vi "总磷总氮通讯.vi"() -> ()   [LabVIEW 2022 SP3, in "斯坦道氨氮.lvlib"]
uses:
  <vilib>/Plasmionique/MB Master/MB_Master_Serial/MB_Master_Serial.lvclass
  C:/Program Files (x86)/National Instruments/LabVIEW 2022/vi.lib/Plasmionique/MB Master/MB_Master/MB_Master.lvclass
  <vilib>/Plasmionique/MB Master/MB_Master_TCP/MB_Master_TCP.lvclass
  <vilib>/Utility/config.llb/Write Key (Boolean).vi
  <vilib>/Utility/config.llb/Write Key (String).vi
  <vilib>/Plasmionique/MB Master/MB_Master/MB_Master.lvclass
  <vilib>/Utility/config.llb/NI_LVConfig.lvlib
  <vilib>/Plasmionique/MB Master/MB Master.lvlib
  <vilib>/ptbypt/NI_PtbyPt.lvlib
panel:
  out "启用":bool=TRUE
  out "氨氮状态告警区":u16[](array[numeric])
  out "氨氮测量数据区":u16[](array[numeric])
  out "COD测量数据区":u16[](array[numeric])
  out "COD状态告警区":u16[](array[numeric])
  out "总氮测量数据区":u16[](array[numeric])
  out "总氮状态告警区":u16[](array[numeric])
  out "总磷状态告警区":u16[](array[numeric])
  out "总磷测量数据区":u16[](array[numeric])
  out "状态告警区":T1 {"告警代码" items=["无告警", "缺试剂告警", "缺水样告警", "缺蒸馏水告警", "缺标液告警", "仪表漏液告警", "标定异常告警", "超量程告警", "加热异常", "低试剂预警", "超上限告警", "超下限告警", "仪表内部其他异常", "滴定异常告警", "电极异常告警", "量程切换告警", "参数设置告警", "PH电极电位异常", "电导率电极异常", "浊度光度异常", "溶解氧电极异常", "溶解氧光强异常", "温度异常告警", "PH异常告警", "溶解氧异常告警", "电导率异常告警", "浊度异常告警", "叶绿素异常告警", "藻密度异常告警", "蓝绿藻异常告警", "ORP异常告警", "氨氮异常告警", "清洁刷异常告警", "SD卡异常告警", "蓝牙异常告警", "Wifi异常告警", "流程异常告警"]; "故障代码" items=["无故障", "电机故障", "温度故障", "通讯故障", "滴定故障"]}
  out "测量数据区":T2 {"单位" items=["ug/L", "mg/L", "ppm", "mg/m3", "cm", "ppb", "ug/m3", "%", "nmol/mol", "umol/mol", "MPN/L", "MPN/100ml", "ng/m3", "NTU", "无量纲", "ms/cm", "us/cm", "℃", "mV", "万个/L"]}
  out "status":bool
  out "关键参数区":T3
  in  "读关键参数区":bool
  in  "读状态告警区":bool
  in  "读测量数据区":bool
  in  "站号":u16(ring) items=["总磷"=1, "氨氮"=3]
  in  "停止":bool
  in  "启动":bool
  in  "控制命令":u16(ring) items=["启动测量"=1, "标样核查"=2, "零点核查"=3, "跨度核查"=4, "空白测试"=5, "平行样测试"=6, "加标回收"=7, "空白校准"=8, "标样校准"=9, "初始化（清洗）"=10, "停止测试"=11, "仪器重启"=12, "校时"=13, "模式设置"=14, "测量间隔设置"=15]
  in  "控制命令参数":u16[](array[numeric]) format="%04xH"
  in  "VISA Resource":refnum<visa-resource-name>
  in  "启用模块":bool
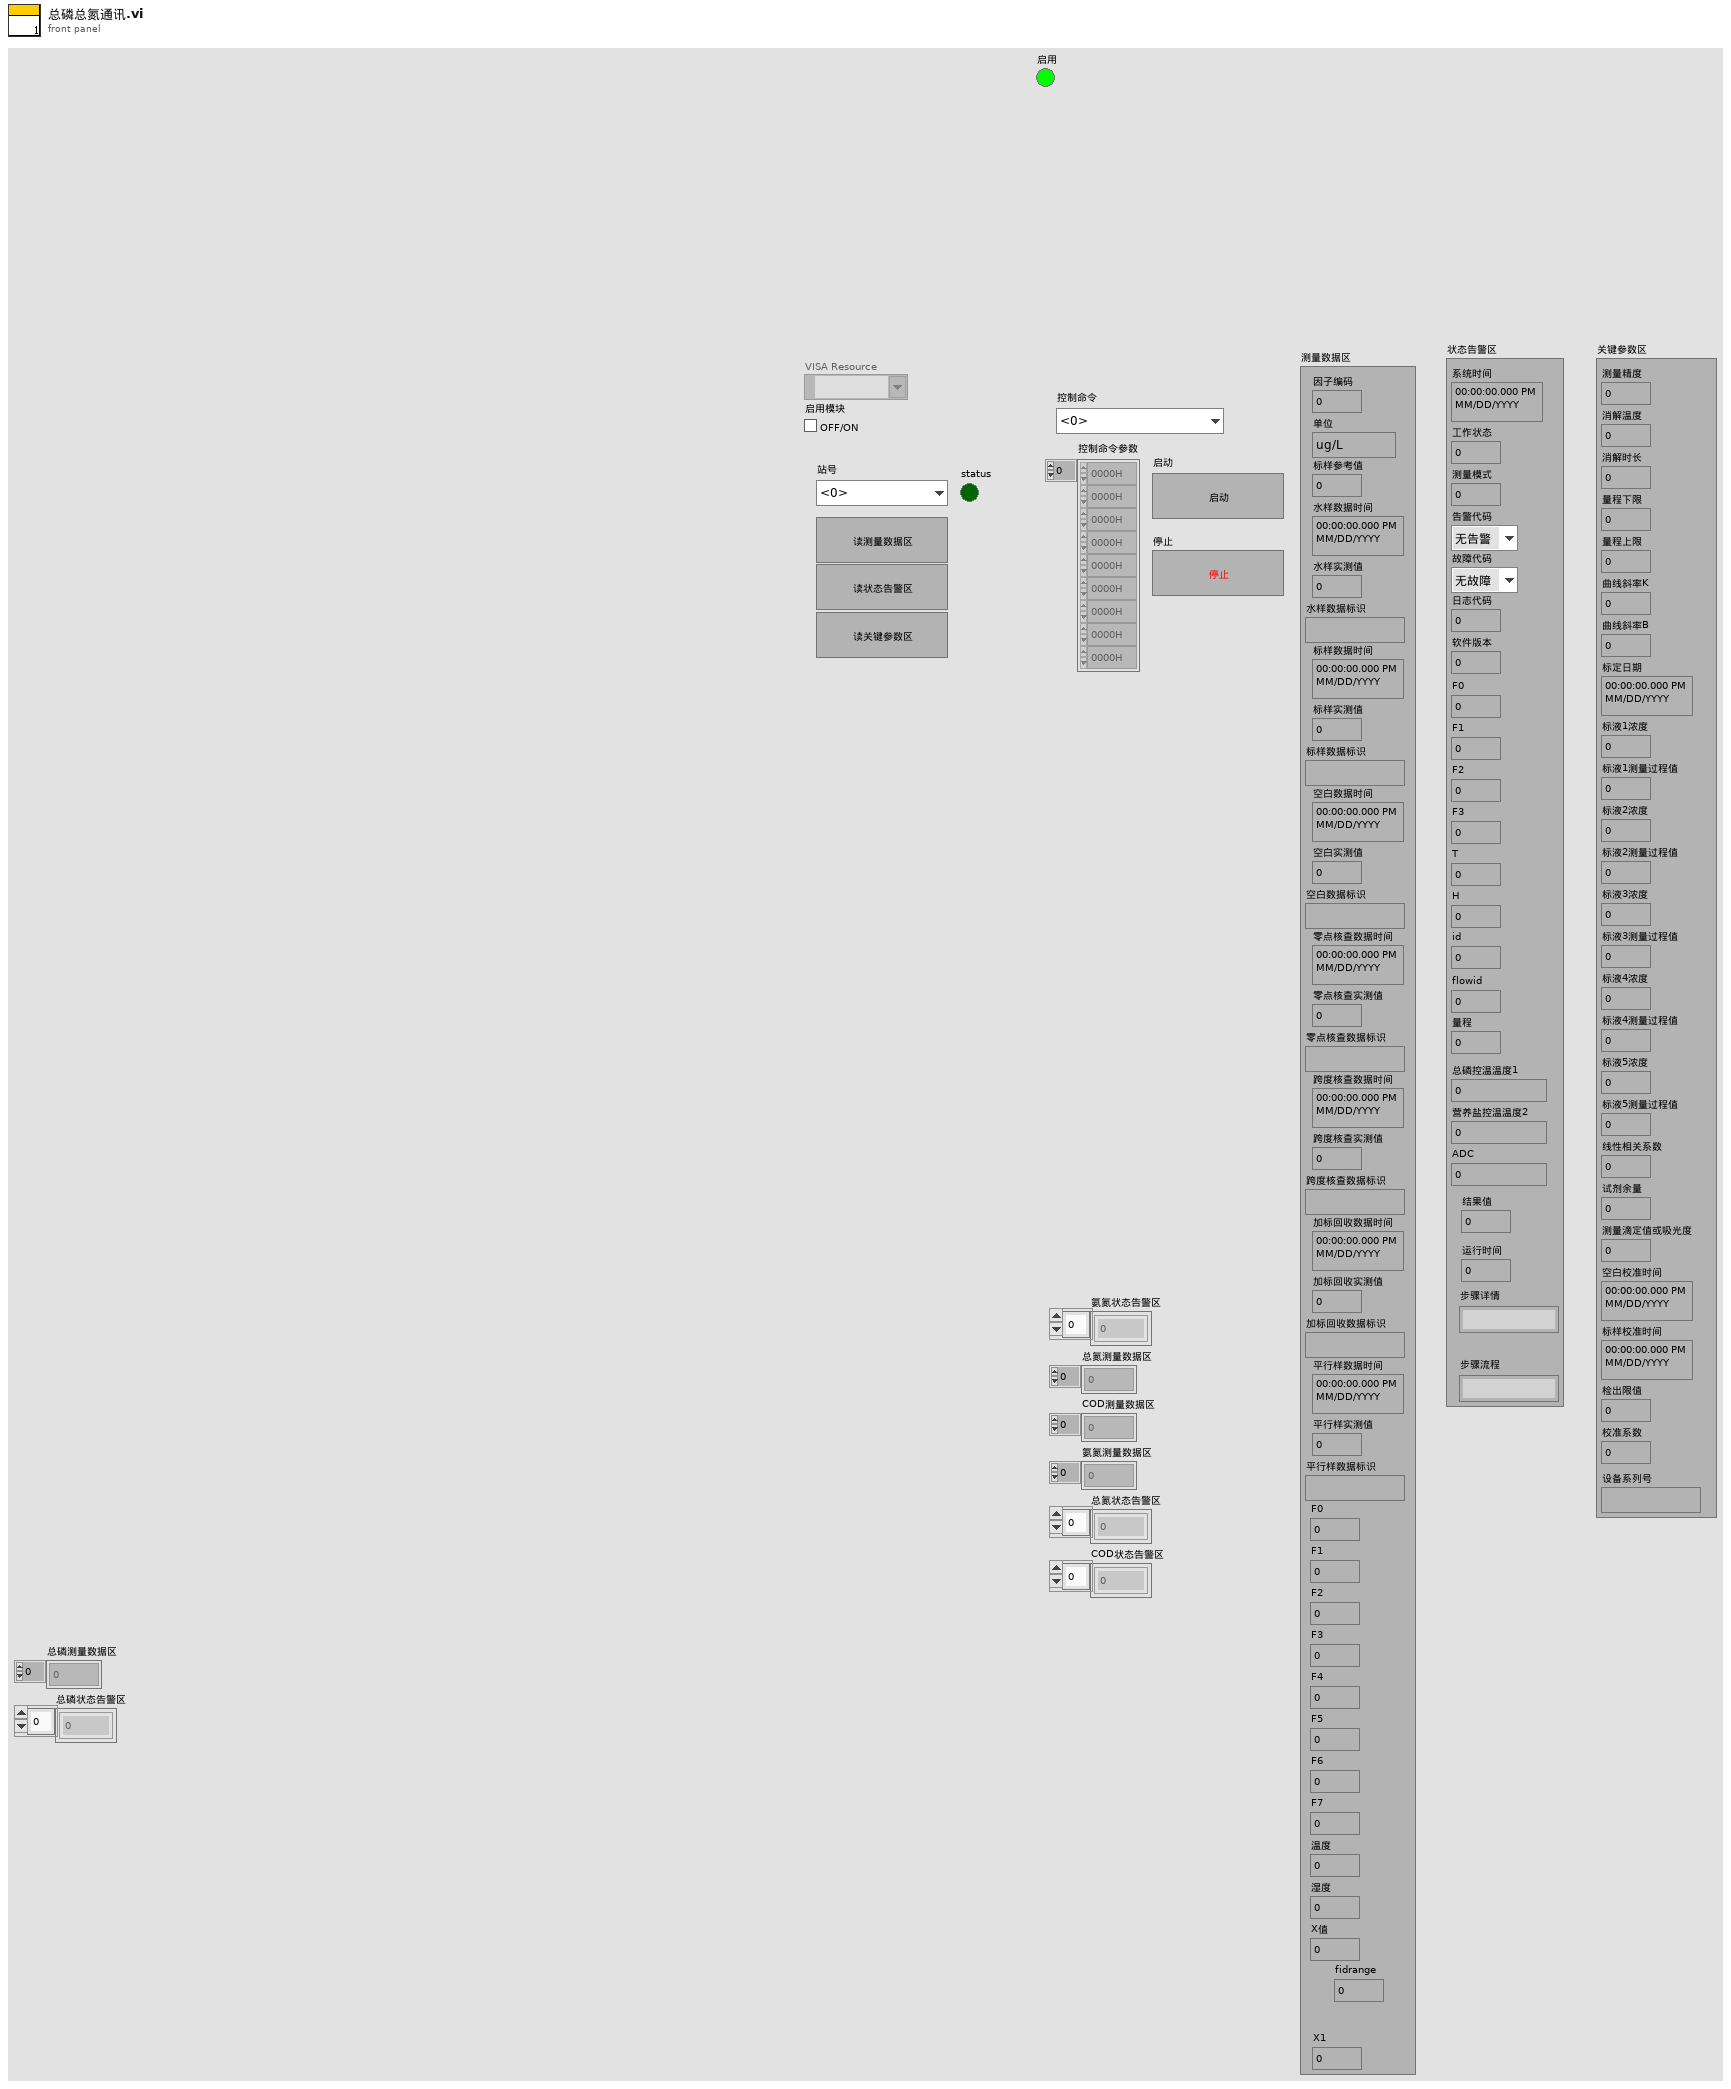
[diagram p1: front panel]
types:
  T1 = cluster{"系统时间":timestamp, "工作状态":u16, "测量模式":u16, "告警代码":u16, "故障代码":u16, "日志代码":u16, "软件版本":u16, "F0":sgl, "F1":sgl, "F2":sgl, "F3":sgl, "T":sgl, "H":sgl, "id":u16, "flowid":u16, "量程":u16, "总磷控温温度1":sgl, "营养盐控温温度2":sgl, "ADC":sgl, "结果值":sgl, "运行时间":u16, "步骤详情":string, "步骤流程":string}
  T2 = cluster{"因子编码":u32, "单位":u16, "标样参考值":sgl, "水样数据时间":timestamp, "水样实测值":sgl, "水样数据标识":string, "标样数据时间":timestamp, "标样实测值":sgl, "标样数据标识":string, "空白数据时间":timestamp, "空白实测值":sgl, "空白数据标识":string, "零点核查数据时间":timestamp, "零点核查实测值":sgl, "零点核查数据标识":string, "跨度核查数据时间":timestamp, "跨度核查实测值":sgl, "跨度核查数据标识":string, "加标回收数据时间":timestamp, "加标回收实测值":sgl, "加标回收数据标识":string, "平行样数据时间":timestamp, "平行样实测值":sgl, "平行样数据标识":string, "F0":sgl, "F1":sgl, "F2":sgl, "F3":sgl, "F4":sgl, "F5":sgl, "F6":sgl, "F7":sgl, "温度":sgl, "湿度":sgl, "X值":sgl, "fidrange":u16, "X1":sgl}
  T3 = cluster{"测量精度":u16, "消解温度":u16, "消解时长":u16, "量程下限":sgl, "量程上限":sgl, "曲线斜率K":sgl, "曲线斜率B":sgl, "标定日期":timestamp, "标液1浓度":sgl, "标液1测量过程值":sgl, "标液2浓度":sgl, "标液2测量过程值":sgl, "标液3浓度":sgl, "标液3测量过程值":sgl, "标液4浓度":sgl, "标液4测量过程值":sgl, "标液5浓度":sgl, "标液5测量过程值":sgl, "线性相关系数":sgl, "试剂余量":u32, "测量滴定值或吸光度":sgl, "空白校准时间":timestamp, "标样校准时间":timestamp, "检出限值":sgl, "校准系数":sgl, "设备系列号":string}
  T4 = cluster{"系统时间":timestamp, "工作状态":u16, "测量模式":enum16{"待机", "连续模式", "周期模式", "定点模式", "受控模式", "手动模式"}, "告警代码":u16, "故障代码":u16, "日志代码":u16, "软件版本":u16, "F0":sgl, "F1":sgl, "F2":sgl, "F3":sgl, "T":sgl, "H":sgl, "id":u16, "flowid":u16, "量程":u16, "总磷控温温度1":sgl, "营养盐控温温度2":sgl, "ADC":sgl}
  T5 = cluster{"因子编码":u32, "单位":u16, "标样参考值":sgl, "水样数据时间":timestamp, "水样实测值":sgl, "水样数据标识":string, "标样数据时间":timestamp, "标样实测值":sgl, "标样数据标识":string, "空白数据时间":timestamp, "空白实测值":sgl, "空白数据标识":string, "零点核查数据时间":timestamp, "零点核查实测值":sgl, "零点核查数据标识":string, "跨度核查数据时间":timestamp, "跨度核查实测值":sgl, "跨度核查数据标识":string, "加标回收数据时间":timestamp, "加标回收实测值":sgl, "加标回收数据标识":string, "平行样数据时间":timestamp, "平行样实测值":sgl, "平行样数据标识":string, "F0":sgl, "F1":sgl, "F2":sgl, "F3":sgl, "F4":sgl, "F5":sgl, "F6":sgl, "F7":sgl, "温度":sgl, "湿度":sgl, "X值":sgl, "fidrange":u16, "X1值":sgl}
  T6 = cluster{"测量精度":u16, "消解温度":u16, "消解时长":u16, "量程下限":sgl, "量程上限":sgl, "曲线斜率K":sgl, "曲线斜率B":sgl, "标定日期":timestamp, "标液1浓度":sgl, "标液1测量过程值":sgl, "标液2浓度":sgl, "标液2测量过程值":sgl, "标液3浓度":sgl, "标液3测量过程值":sgl, "标液4浓度":sgl, "标液4测量过程值":sgl, "标液5浓度":sgl, "标液5测量过程值":sgl, "线性相关系数":sgl, "试剂余量":u32, "测量滴定值或吸光度":sgl, "空白校准时间":timestamp, "标样校准时间":timestamp, "检出限值":sgl, "校准系数":sgl, "设备系列号":string}[]
  T7 = cluster{"系统时间":timestamp, "工作状态":u16, "测量模式":enum16{"待机", "连续模式", "周期模式", "定点模式", "受控模式", "手动模式"}, "告警代码":u16, "故障代码":u16, "日志代码":u16, "软件版本":u16, "F0":sgl, "F1":sgl, "F2":sgl, "F3":sgl, "T":sgl, "H":sgl, "id":u16, "flowid":u16, "量程":u16, "总磷控温温度1":sgl, "营养盐控温温度2":sgl, "ADC":sgl}[]
  T8 = cluster{"因子编码":u32, "单位":u16, "标样参考值":sgl, "水样数据时间":timestamp, "水样实测值":sgl, "水样数据标识":string, "标样数据时间":timestamp, "标样实测值":sgl, "标样数据标识":string, "空白数据时间":timestamp, "空白实测值":sgl, "空白数据标识":string, "零点核查数据时间":timestamp, "零点核查实测值":sgl, "零点核查数据标识":string, "跨度核查数据时间":timestamp, "跨度核查实测值":sgl, "跨度核查数据标识":string, "加标回收数据时间":timestamp, "加标回收实测值":sgl, "加标回收数据标识":string, "平行样数据时间":timestamp, "平行样实测值":sgl, "平行样数据标识":string, "F0":sgl, "F1":sgl, "F2":sgl, "F3":sgl, "F4":sgl, "F5":sgl, "F6":sgl, "F7":sgl, "温度":sgl, "湿度":sgl, "X值":sgl, "fidrange":u16, "X1值":sgl}[]
  T9 = enum16{"", "CODMn", "PH", "氨氮", "总氮", "总磷", "CODCr", "电导率", "水温", "溶解氧", "浊度", "叶绿素", "藻密度", "ORP"}
  T10 = typedef "CODCr交互.ctl" = cluster{"状态告警区":cluster{"系统时间":timestamp, "工作状态":u16, "测量模式":enum16{"待机", "连续模式", "周期模式", "定点模式", "受控模式", "手动模式"}, "告警代码":u16, "故障代码":u16, "日志代码":u16, "软件版本":u16, "F0":sgl, "F1":sgl, "F2":sgl, "F3":sgl, "T":sgl, "H":sgl, "id":u16, "flowid":u16, "量程":u16, "总磷控温温度1":sgl, "营养盐控温温度2":sgl, "ADC":sgl}, "平台试剂余量百分比":sgl, "关键参数":cluster{"测量量程":dbl, "测量精度":dbl, "测量间隔":dbl, "消解温度":dbl, "消解时长":dbl, "空白校准时间":timestamp, "曲线截距":dbl, "曲线斜率":dbl, "测量检出限":dbl, "测量信号值":dbl, "线性相关系数":dbl, "二次多项式系数":dbl, "标样校准时间":timestamp, "稀释倍数":dbl, "三项式系数":dbl, "空白标定系数":dbl, "量程系数":dbl, "F0/ORPA":dbl, "F1/ORPB":dbl, "F2/ORPK":dbl, "F3":dbl, "F4":dbl, "F5":dbl, "F6":dbl, "F7":dbl, "X0/滴定数":dbl, "量程":dbl}, "关键参数改变":bool, "校准信息":cluster{"低标液1浓度":dbl, "低标液1信号值":dbl, "低标液1启用":u16, "低标液2浓度":dbl, "低标液2信号值":dbl, "低标液2启用":u16, "低标液3浓度":dbl, "低标液3信号值":dbl, "低标液3启用":u16, "低标液4浓度":dbl, "低标液4信号值":dbl, "低标液4启用":u16, "低标液5浓度":dbl, "低标液5信号值":dbl, "低标液5启用":u16, "高标液1浓度":dbl, "高标液1信号值":dbl, "高标液1启用":u16, "高标液2浓度":dbl, "高标液2信号值":dbl, "高标液2启用":u16, "高标液3浓度":dbl, "高标液3信号值":dbl, "高标液3启用":u16, "高标液4浓度":dbl, "高标液4信号值":dbl, "高标液4启用":u16, "高标液5浓度":dbl, "高标液5信号值":dbl, "高标液5启用":u16, "低斜率":dbl, "低截距":dbl, "低二次多项式系数":dbl, "低线性相关系数":dbl, "高斜率":dbl, "高截距":dbl, "高二次多项式系数":dbl, "高线性相关系数":dbl}, "校准信息改变":bool, "固件版本号":string}
  T11 = typedef "总磷交互.ctl" = cluster{"状态告警区":cluster{"系统时间":timestamp, "工作状态":u16, "测量模式":enum16{"待机", "连续模式", "周期模式", "定点模式", "受控模式", "手动模式"}, "告警代码":u16, "故障代码":u16, "日志代码":u16, "软件版本":u16, "F0":sgl, "F1":sgl, "F2":sgl, "F3":sgl, "T":sgl, "H":sgl, "id":u16, "flowid":u16, "量程":u16, "总磷控温温度1":sgl, "营养盐控温温度2":sgl, "ADC":sgl}, "平台试剂余量百分比":sgl, "关键参数":cluster{"测量量程":dbl, "测量精度":dbl, "测量间隔":dbl, "消解温度":dbl, "消解时长":dbl, "空白校准时间":timestamp, "曲线截距":dbl, "曲线斜率":dbl, "测量检出限":dbl, "测量信号值":dbl, "线性相关系数":dbl, "二次多项式系数":dbl, "标样校准时间":timestamp, "稀释倍数":dbl, "三项式系数":dbl, "空白标定系数":dbl, "量程系数":dbl, "F0/ORPA":dbl, "F1/ORPB":dbl, "F2/ORPK":dbl, "F3":dbl, "F4":dbl, "F5":dbl, "F6":dbl, "F7":dbl, "X0/滴定数":dbl, "量程":dbl}, "关键参数改变":bool, "校准信息":cluster{"低标液1浓度":dbl, "低标液1信号值":dbl, "低标液1启用":u16, "低标液2浓度":dbl, "低标液2信号值":dbl, "低标液2启用":u16, "低标液3浓度":dbl, "低标液3信号值":dbl, "低标液3启用":u16, "低标液4浓度":dbl, "低标液4信号值":dbl, "低标液4启用":u16, "低标液5浓度":dbl, "低标液5信号值":dbl, "低标液5启用":u16, "高标液1浓度":dbl, "高标液1信号值":dbl, "高标液1启用":u16, "高标液2浓度":dbl, "高标液2信号值":dbl, "高标液2启用":u16, "高标液3浓度":dbl, "高标液3信号值":dbl, "高标液3启用":u16, "高标液4浓度":dbl, "高标液4信号值":dbl, "高标液4启用":u16, "高标液5浓度":dbl, "高标液5信号值":dbl, "高标液5启用":u16, "低斜率":dbl, "低截距":dbl, "低二次多项式系数":dbl, "低线性相关系数":dbl, "高斜率":dbl, "高截距":dbl, "高二次多项式系数":dbl, "高线性相关系数":dbl}, "校准信息改变":bool, "固件版本号":string}
  T12 = typedef "总氮交互.ctl" = cluster{"状态告警区":cluster{"系统时间":timestamp, "工作状态":u16, "测量模式":enum16{"待机", "连续模式", "周期模式", "定点模式", "受控模式", "手动模式"}, "告警代码":u16, "故障代码":u16, "日志代码":u16, "软件版本":u16, "F0":sgl, "F1":sgl, "F2":sgl, "F3":sgl, "T":sgl, "H":sgl, "id":u16, "flowid":u16, "量程":u16, "总磷控温温度1":sgl, "营养盐控温温度2":sgl, "ADC":sgl}, "平台试剂余量百分比":sgl, "关键参数":cluster{"测量量程":dbl, "测量精度":dbl, "测量间隔":dbl, "消解温度":dbl, "消解时长":dbl, "空白校准时间":timestamp, "曲线截距":dbl, "曲线斜率":dbl, "测量检出限":dbl, "测量信号值":dbl, "线性相关系数":dbl, "二次多项式系数":dbl, "标样校准时间":timestamp, "稀释倍数":dbl, "三项式系数":dbl, "空白标定系数":dbl, "量程系数":dbl, "F0/ORPA":dbl, "F1/ORPB":dbl, "F2/ORPK":dbl, "F3":dbl, "F4":dbl, "F5":dbl, "F6":dbl, "F7":dbl, "X0/滴定数":dbl, "量程":dbl}, "关键参数改变":bool, "校准信息":cluster{"低标液1浓度":dbl, "低标液1信号值":dbl, "低标液1启用":u16, "低标液2浓度":dbl, "低标液2信号值":dbl, "低标液2启用":u16, "低标液3浓度":dbl, "低标液3信号值":dbl, "低标液3启用":u16, "低标液4浓度":dbl, "低标液4信号值":dbl, "低标液4启用":u16, "低标液5浓度":dbl, "低标液5信号值":dbl, "低标液5启用":u16, "高标液1浓度":dbl, "高标液1信号值":dbl, "高标液1启用":u16, "高标液2浓度":dbl, "高标液2信号值":dbl, "高标液2启用":u16, "高标液3浓度":dbl, "高标液3信号值":dbl, "高标液3启用":u16, "高标液4浓度":dbl, "高标液4信号值":dbl, "高标液4启用":u16, "高标液5浓度":dbl, "高标液5信号值":dbl, "高标液5启用":u16, "低斜率":dbl, "低截距":dbl, "低二次多项式系数":dbl, "低线性相关系数":dbl, "高斜率":dbl, "高截距":dbl, "高二次多项式系数":dbl, "高线性相关系数":dbl}, "校准信息改变":bool, "固件版本号":string}
  T13 = typedef "氨氮交互.ctl" = cluster{"状态告警区":cluster{"系统时间":timestamp, "工作状态":u16, "测量模式":enum16{"待机", "连续模式", "周期模式", "定点模式", "受控模式", "手动模式"}, "告警代码":u16, "故障代码":u16, "日志代码":u16, "软件版本":u16, "F0":sgl, "F1":sgl, "F2":sgl, "F3":sgl, "T":sgl, "H":sgl, "id":u16, "flowid":u16, "量程":u16, "总磷控温温度1":sgl, "营养盐控温温度2":sgl, "ADC":sgl}, "平台试剂余量百分比":sgl, "关键参数":cluster{"测量量程":dbl, "测量精度":dbl, "测量间隔":dbl, "消解温度":dbl, "消解时长":dbl, "空白校准时间":timestamp, "曲线截距":dbl, "曲线斜率":dbl, "测量检出限":dbl, "测量信号值":dbl, "线性相关系数":dbl, "二次多项式系数":dbl, "标样校准时间":timestamp, "稀释倍数":dbl, "三项式系数":dbl, "空白标定系数":dbl, "量程系数":dbl, "F0/ORPA":dbl, "F1/ORPB":dbl, "F2/ORPK":dbl, "F3":dbl, "F4":dbl, "F5":dbl, "F6":dbl, "F7":dbl, "X0/滴定数":dbl, "量程":dbl}, "关键参数改变":bool, "校准信息":cluster{"低标液1浓度":dbl, "低标液1信号值":dbl, "低标液1启用":u16, "低标液2浓度":dbl, "低标液2信号值":dbl, "低标液2启用":u16, "低标液3浓度":dbl, "低标液3信号值":dbl, "低标液3启用":u16, "低标液4浓度":dbl, "低标液4信号值":dbl, "低标液4启用":u16, "低标液5浓度":dbl, "低标液5信号值":dbl, "低标液5启用":u16, "高标液1浓度":dbl, "高标液1信号值":dbl, "高标液1启用":u16, "高标液2浓度":dbl, "高标液2信号值":dbl, "高标液2启用":u16, "高标液3浓度":dbl, "高标液3信号值":dbl, "高标液3启用":u16, "高标液4浓度":dbl, "高标液4信号值":dbl, "高标液4启用":u16, "高标液5浓度":dbl, "高标液5信号值":dbl, "高标液5启用":u16, "低斜率":dbl, "低截距":dbl, "低二次多项式系数":dbl, "低线性相关系数":dbl, "高斜率":dbl, "高截距":dbl, "高二次多项式系数":dbl, "高线性相关系数":dbl}, "校准信息改变":bool, "固件版本号":string}
  T14 = typedef "NI_LVConfig.lvlib/Config Data RefNum.ctl" = refnum<k1>
  T15 = enum8{"Enabled", "Disabled", "Disabled and Grayed Out"}
  T16 = cluster{"baud rate (bps)":u32, "stop bits":u16, "parity":u16, "flow control":u16, "timeout":u32, "retries":i32}
  T17 = typedef "工况数据.ctl" = cluster{"time":string, "data":cluster{"ups":cluster{"ups":cluster{"input_voltage":ext, "input_frequency":ext, "output_voltage":ext, "output_current":ext, "output_frequency":ext, "output_active_power":ext, "output_apparent_power":ext, "load_rate":ext, "cabinet_temperature":ext, "battery_voltage":ext, "remaining_battery_capacity":ext, "power_on_status":string, "power_supply_mode":string, "fault":bool, "battery_low_voltage":bool, "mains_supply_abnormality":bool}, "启用":bool}, "air_conditioner":cluster{"air_conditioner":cluster{"cabinet_temperature":ext, "air_supply_temperature":ext, "voltage":ext, "current":ext, "compressor_status":string, "Internal_fan_status":string, "external_fan_status":string, "heating_state":string, "refrigeration_state":bool, "high_temperature_alarm":bool, "low_temperature_alarm":bool, "heater_fault":bool, "temperature_sensor_fault":bool, "high_voltage_alarm":bool, "low_voltage_alarm":bool, "refrigeration_start_point":ext, "refrigeration_sensitive_point":ext, "heating_start_point":ext, "heating_sensitive_point":ext, "high_temperature_alarm_point":ext, "low_temperature_alarm_point":ext}, "启用":bool}, "smoke_sensor":cluster{"smoke_sensor":cluster{"trigger_alarm":bool}, "启用":bool}, "water_immersion_sensor":cluster{"water_immersion_sensor":cluster{"trigger_alarm":bool}, "启用":bool}, "temperature_and_humidity_sensor":cluster{"temperature_and_humidity_sensor":cluster{"current_temperature":ext, "current_humidity":ext, "room_temperature_alarm":bool, "humidity_alarm":bool}, "启用":bool}, "gps":cluster{"gps":cluster{"current_longitude":ext, "current_latitude":ext, "launch_longitude":ext, "launch_latitude":ext, "shift_alarm":bool}, "启用":bool}, "solar_controller":cluster{"solar_controller":cluster{"array_voltage":ext, "array_current":ext, "generating_power":ext, "battery_voltage":dbl, "battery_current":ext, "ceiling_voltage":ext, "minimum_voltage":ext, "battery_temperature":ext, "remaining_battery_capacity":ext, "load_voltage":ext, "load_current":ext, "load_power":ext, "equipment_temperature":ext, "accumulated_electricity_consumption_of_the_day":ext, "accumulated_electricity_consumption_of_the_current_month":ext, "accumulated_electricity_consumption_in_the_current_year":ext, "total_accumulated_power_consumption":ext, "accumulated_charging_capacity_of_the_day":ext, "accumulated_charging_amount_of_the_current_month":ext, "accumulated_charging_capacity_of_the_current_year":ext, "total_cumulative_charge":ext}, "启用":bool}, "solar_controller_2":cluster{"solar_controller_2":cluster{"array_voltage":ext, "array_current":ext, "generating_power":ext, "battery_voltage":dbl, "battery_current":ext, "ceiling_voltage":ext, "minimum_voltage":ext, "battery_temperature":ext, "remaining_battery_capacity":ext, "load_voltage":ext, "load_current":ext, "load_power":ext, "equipment_temperature":ext, "accumulated_electricity_consumption_of_the_day":ext, "accumulated_electricity_consumption_of_the_current_month":ext, "accumulated_electricity_consumption_in_the_current_year":ext, "total_accumulated_power_consumption":ext, "accumulated_charging_capacity_of_the_day":ext, "accumulated_charging_amount_of_the_current_month":ext, "accumulated_charging_capacity_of_the_current_year":ext, "total_cumulative_charge":ext}, "启用":bool}, "NH3":cluster{"NH3":cluster{"F0":ext, "F1":ext, "syringe_temperature":ext, "alarm_step":dbl, "X0":ext}, "启用":bool}, "TP":cluster{"TP":cluster{"F0":ext, "F1":ext, "F2":ext, "F3":ext, "digestion_temperature":ext, "constant_temperature":ext, "syringe_temperature":ext, "alarm_step":dbl, "X0":ext}, "启用":bool}, "TN":cluster{"TN":cluster{"F0":ext, "F1":ext, "F2":ext, "F3":ext, "F4":ext, "F5":ext, "F6":ext, "F7":ext, "digestion_temperature":ext, "constant_temperature":ext, "syringe_temperature":ext, "alarm_step":dbl, "X0":ext}, "启用":bool}, "CODMn":cluster{"CODMn":cluster{"temperature_curve":ext[], "titration_curve":ext[], "F0":ext, "F1":ext, "F2":ext, "F3":ext, "F4":ext, "F5":ext, "A":ext, "B":ext, "K":ext}, "启用":bool}, "CODCr":cluster{"CODCr":cluster{"temperature_curve":ext[], "F0":ext, "F1":ext, "reagent_sensor":ext}, "启用":bool}}}
  T18 = cluster{"系统时间":timestamp, "工作状态":u16, "测量模式":enum16{"待机", "连续模式", "周期模式", "定点模式", "受控模式", "手动模式"}, "告警代码":u16, "故障代码":u16, "日志代码":u16, "软件版本":u16, "F0":sgl, "F1":sgl, "F2":sgl, "F3":sgl, "T":sgl, "H":sgl, "id":u16, "flowid":u16, "量程":u16, "总磷控温温度1":sgl, "营养盐控温温度2":sgl, "ADC":sgl, "结果值":sgl, "运行时间":u16, "步骤详情":string, "步骤流程":string}
  T19 = typedef "斯坦道氨氮.lvlib/关键参数.ctl" = cluster{"测量量程":sgl, "测量检出限":sgl, "测量精度":sgl, "测量间隔":sgl, "消解温度":sgl, "消解时长":sgl, "三项式系数":sgl, "二次多项式系数":sgl, "曲线斜率":sgl, "曲线截距":sgl, "线性相关系数":sgl, "空白校准时间":timestamp, "标样校准时间":timestamp, "测量信号值":sgl, "稀释倍数":sgl, "空白标定系数":sgl, "量程系数":sgl}
  T20 = cluster{"测量精度":u16, "消解温度":u16, "消解时长":u16, "量程下限":sgl, "量程上限":sgl, "曲线斜率K":sgl, "曲线截距B":sgl, "标定日期":timestamp, "标液1浓度":sgl, "标液1测量过程值":sgl, "标液2浓度":sgl, "标液2测量过程值":sgl, "标液3浓度":sgl, "标液3测量过程值":sgl, "标液4浓度":sgl, "标液4测量过程值":sgl, "标液5浓度":sgl, "标液5测量过程值":sgl, "线性相关系数":sgl, "试剂余量":u32, "测量滴定值或吸光度":sgl, "空白校准时间":timestamp, "标样校准时间":timestamp, "检出限值":sgl, "校准系数":sgl, "设备系列号":string}
  T21 = cluster{"测量量程":dbl, "测量精度":dbl, "测量间隔":dbl, "消解温度":dbl, "消解时长":dbl, "空白校准时间":timestamp, "曲线截距":dbl, "曲线斜率":dbl, "测量检出限":dbl, "测量信号值":dbl, "线性相关系数":dbl, "二次多项式系数":dbl, "标样校准时间":timestamp, "稀释倍数":dbl, "三项式系数":dbl, "空白标定系数":dbl, "量程系数":dbl, "F0/ORPA":dbl, "F1/ORPB":dbl, "F2/ORPK":dbl, "F3":dbl, "F4":dbl, "F5":dbl, "F6":dbl, "F7":dbl, "X0/滴定数":dbl, "量程":dbl}
  T22 = cluster{"低标液1浓度":dbl, "低标液1信号值":dbl, "低标液1启用":u16, "低标液2浓度":dbl, "低标液2信号值":dbl, "低标液2启用":u16, "低标液3浓度":dbl, "低标液3信号值":dbl, "低标液3启用":u16, "低标液4浓度":dbl, "低标液4信号值":dbl, "低标液4启用":u16, "低标液5浓度":dbl, "低标液5信号值":dbl, "低标液5启用":u16, "高标液1浓度":dbl, "高标液1信号值":dbl, "高标液1启用":u16, "高标液2浓度":dbl, "高标液2信号值":dbl, "高标液2启用":u16, "高标液3浓度":dbl, "高标液3信号值":dbl, "高标液3启用":u16, "高标液4浓度":dbl, "高标液4信号值":dbl, "高标液4启用":u16, "高标液5浓度":dbl, "高标液5信号值":dbl, "高标液5启用":u16, "低斜率":dbl, "低截距":dbl, "低二次多项式系数":dbl, "低线性相关系数":dbl, "高斜率":dbl, "高截距":dbl, "高二次多项式系数":dbl, "高线性相关系数":dbl}
  T23 = typedef "操作日志字段定义.ctl" = cluster{"时间":timestamp, "参数":string, "日志信息":string, "流程参数":string}
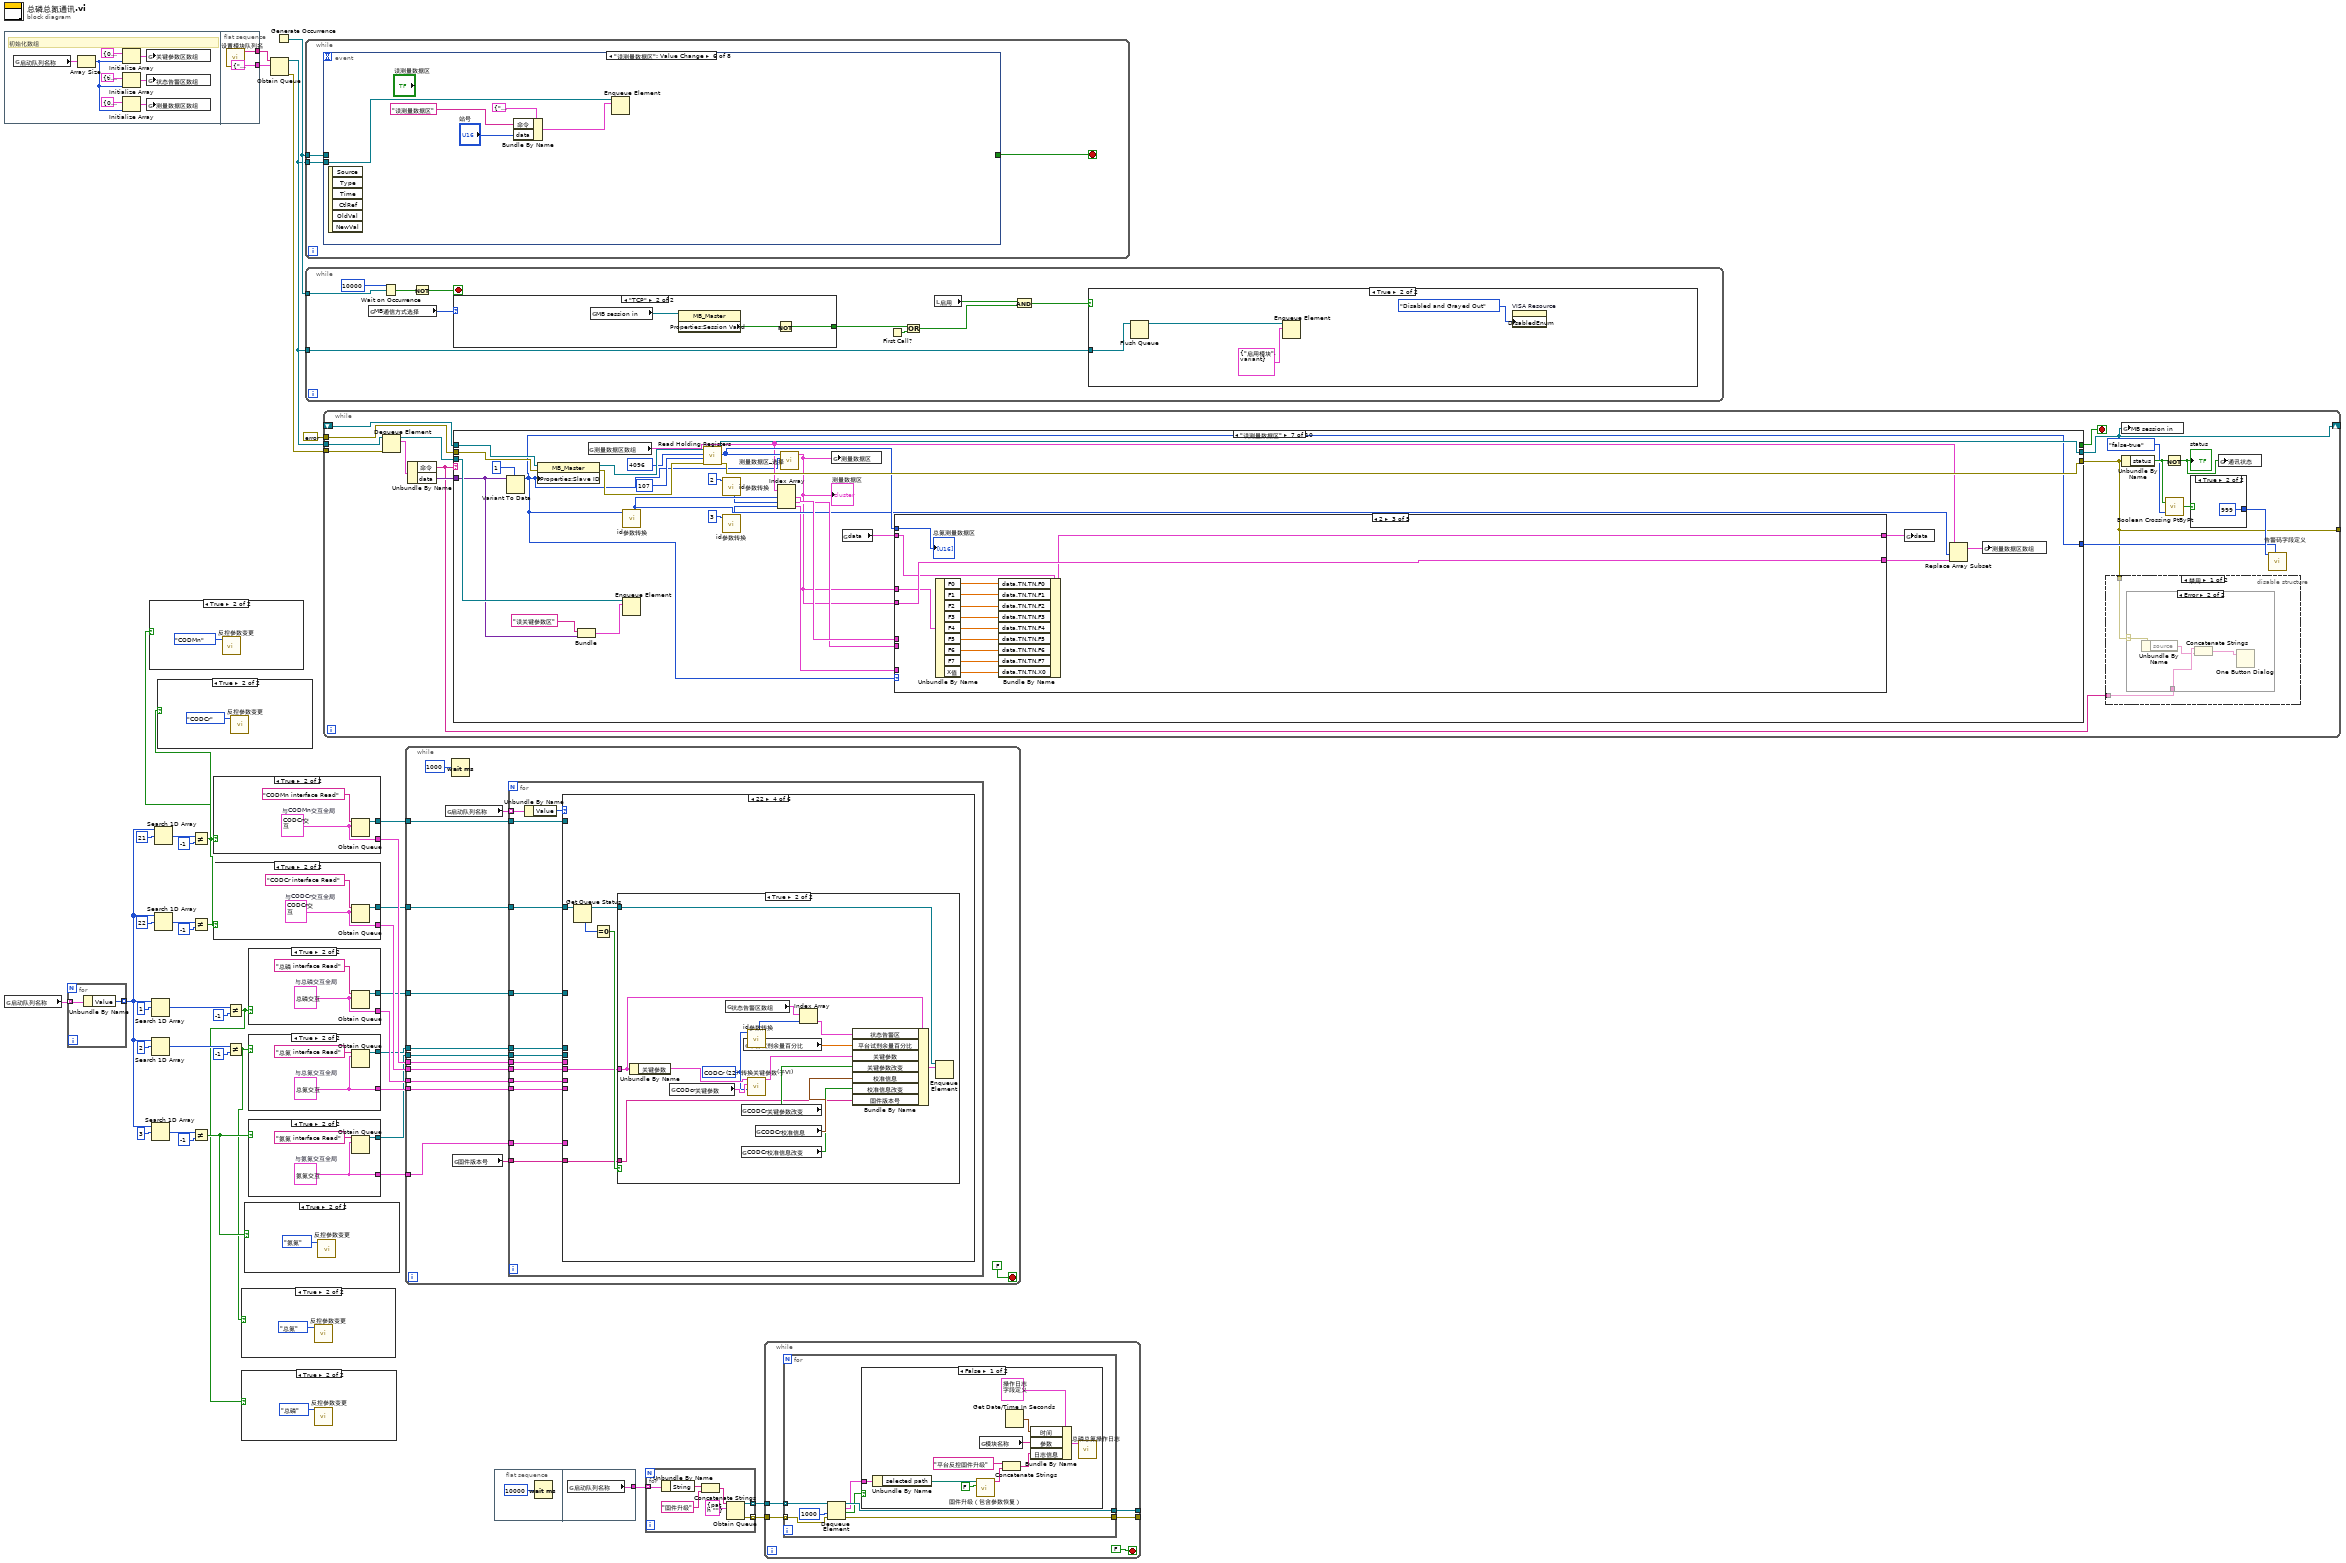
[diagram p0: block diagram]
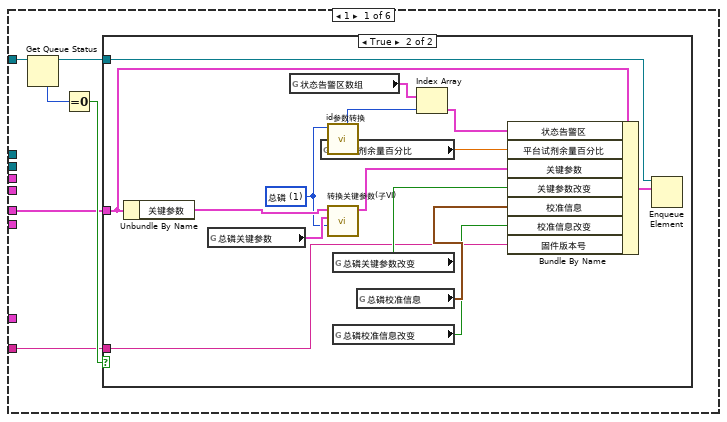
[diagram p13: hidden frame]
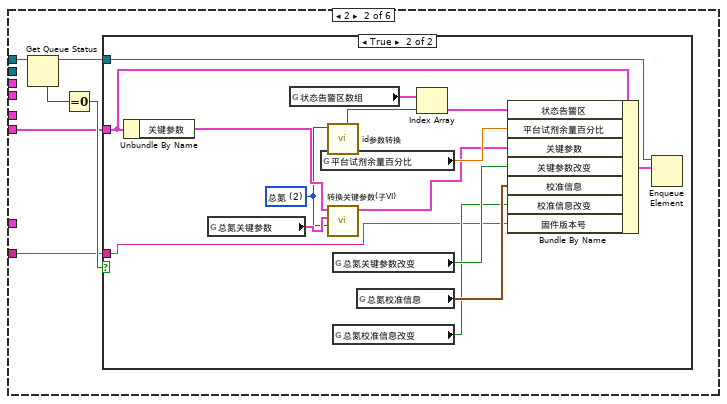
[diagram p15: hidden frame]
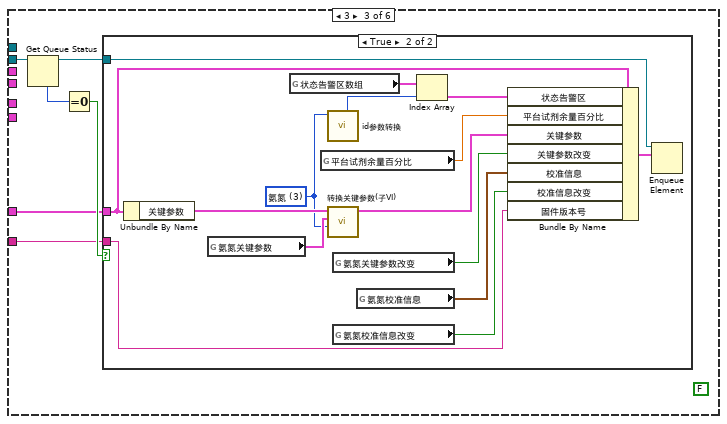
[diagram p17: hidden frame]
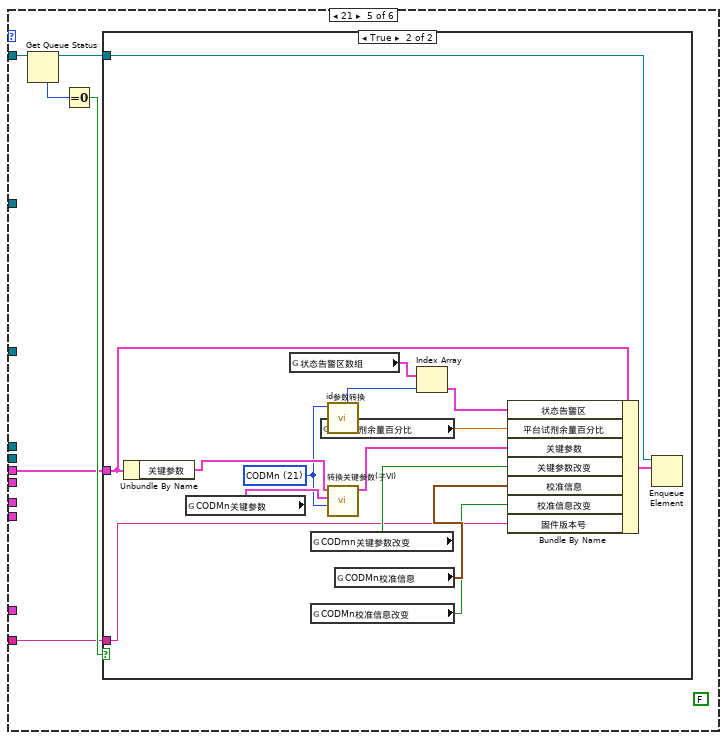
[diagram p20: hidden frame]
diagram:
  n1 = flat-sequence {
    tunnel: [cluster{"命令":string, "data":variant} {"命令"="", "data"=variant}] -> w41
    tunnel: [w50] -> w36
    frame #0 {
      # "初始化数组"
      n2 = global read "model config var.vi" "启动队列名称"() -> (w43:cluster{"String":string, "Value":u16}[])
      n3 = Array Size(array=w43) -> (size(s)=w42:i32)
      n4 = Initialize Array(T3 {"测量精度"=0, "消解温度"=0, "消解时长"=0, "量程下限"=0.0, "量程上限"=0.0, "曲线斜率K"=0.0, "曲线斜率B"=0.0, "标定日期"=timestamp(0 s since 1904-01-01), "标液1浓度"=0.0, "标液1测量过程值"=0.0, "标液2浓度"=0.0, "标液2测量过程值"=0.0, "标液3浓度"=0.0, "标液3测量过程值"=0.0, "标液4浓度"=0.0, "标液4测量过程值"=0.0, "标液5浓度"=0.0, "标液5测量过程值"=0.0, "线性相关系数"=0.0, "试剂余量"=0, "测量滴定值或吸光度"=0.0, "空白校准时间"=timestamp(0 s since 1904-01-01), "标样校准时间"=timestamp(0 s since 1904-01-01), "检出限值"=0.0, "校准系数"=0.0, "设备系列号"=""} ("关键参数区"), w42) -> (w47:T6)
      n5 = Initialize Array(T4 {"系统时间"=timestamp(0 s since 1904-01-01), "工作状态"=0, "测量模式"=enum."待机", "告警代码"=0, "故障代码"=0, "日志代码"=0, "软件版本"=0, "F0"=0.0, "F1"=0.0, "F2"=0.0, "F3"=0.0, "T"=0.0, "H"=0.0, "id"=0, "flowid"=0, "量程"=0, "总磷控温温度1"=0.0, "营养盐控温温度2"=0.0, "ADC"=0.0} ("状态告警区"), w42) -> (w46:T7)
      n6 = Initialize Array(T5 {"因子编码"=0, "单位"=0, "标样参考值"=0.0, "水样数据时间"=timestamp(0 s since 1904-01-01), "水样实测值"=0.0, "水样数据标识"="", "标样数据时间"=timestamp(0 s since 1904-01-01), "标样实测值"=0.0, "标样数据标识"="", "空白数据时间"=timestamp(0 s since 1904-01-01), "空白实测值"=0.0, "空白数据标识"="", "零点核查数据时间"=timestamp(0 s since 1904-01-01), "零点核查实测值"=0.0, "零点核查数据标识"="", "跨度核查数据时间"=timestamp(0 s since 1904-01-01), "跨度核查实测值"=0.0, "跨度核查数据标识"="", "加标回收数据时间"=timestamp(0 s since 1904-01-01), "加标回收实测值"=0.0, "加标回收数据标识"="", "平行样数据时间"=timestamp(0 s since 1904-01-01), "平行样实测值"=0.0, "平行样数据标识"="", "F0"=0.0, "F1"=0.0, "F2"=0.0, "F3"=0.0, "F4"=0.0, "F5"=0.0, "F6"=0.0, "F7"=0.0, "温度"=0.0, "湿度"=0.0, "X值"=0.0, "fidrange"=0, "X1值"=0.0} ("测量数据区"), w42) -> (w49:T8)
      n7 = global write "VAR总磷总氮全局变量.vi" "关键参数区数组"(w47) -> ()
      n8 = global write "VAR总磷总氮全局变量.vi" "状态告警区数组"(w46) -> ()
      n9 = global write "VAR总磷总氮全局变量.vi" "测量数据区数组"(w49) -> ()
    }
    frame #1 {
      n10 = call "设置模块队列名.vi"() -> ("Msg"=w50:string)  [unwired: 5 in]
    }
  }
  n11 = global read "model config var.vi" "启动队列名称"() -> (w25:cluster{"String":string, "Value":u16}[])
  n12 = for {
    tunnel: w25 -> [w53] mode=indexing
    tunnel: [w52] -> w9 mode=indexing
    n13 = Unbundle By Name(w53) -> ("Value"=w52:u16)
  }
  n14 = Search 1D Array(1D array=w9, element=u16 1 ("元素")) -> (index of element=w17:i32)  [unwired: 1 in]
  n15 = Search 1D Array(1D array=w9, element=u16 2 ("元素")) -> (index of element=w14:i32)  [unwired: 1 in]
  n16 = Search 1D Array(1D array=w9, element=u16 3 ("元素")) -> (index of element=w11:i32)  [unwired: 1 in]
  n17 = Search 1D Array(1D array=w9, element=u16 21 ("元素")) -> (index of element=w23:i32)  [unwired: 1 in]
  n18 = Search 1D Array(1D array=w9, element=u16 22 ("元素")) -> (index of element=w20:i32)  [unwired: 1 in]
  n19 = Not Equal?(x=w23, y=-1) -> (x != y?=w1:bool)
  n20 = case shown="True" w1 {
    frame False {
    }
    frame True {
      n21 = call "反控参数变更.vi"("设置参数"=T9."CODMn") -> ()  [unwired: 11 in]
    }
  }
  n22 = Not Equal?(x=w20, y=-1) -> (x != y?=w2:bool)
  n23 = case shown="True" w2 {
    frame False {
    }
    frame True {
      n24 = call "反控参数变更.vi"("设置参数"=T9."CODCr") -> ()  [unwired: 11 in]
    }
  }
  n25 = Not Equal?(x=w11, y=-1) -> (x != y?=w5:bool)
  n26 = case shown="True" w1 {
    tunnel: [_ w57] -> w35
    tunnel: [_ w56] -> w34
    frame False {
    }
    frame True {
      w56 = T10 {"状态告警区"={"系统时间"=timestamp(0 s since 1904-01-01), "工作状态"=0, "测量模式"=enum."待机", "告警代码"=0, "故障代码"=0, "日志代码"=0, "软件版本"=0, "F0"=0.0, "F1"=0.0, "F2"=0.0, "F3"=0.0, "T"=0.0, "H"=0.0, "id"=0, "flowid"=0, "量程"=0, "总磷控温温度1"=0.0, "营养盐控温温度2"=0.0, "ADC"=0.0}, "平台试剂余量百分比"=0.0, "关键参数"={"测量量程"=0.0, "测量精度"=0.0, "测量间隔"=0.0, "消解温度"=0.0, "消解时长"=0.0, "空白校准时间"=timestamp(0 s since 1904-01-01), "曲线截距"=0.0, "曲线斜率"=0.0, "测量检出限"=0.0, "测量信号值"=0.0, "线性相关系数"=0.0, "二次多项式系数"=0.0, "标样校准时间"=timestamp(0 s since 1904-01-01), "稀释倍数"=0.0, "三项式系数"=0.0, "空白标定系数"=0.0, "量程系数"=0.0, "F0/ORPA"=0.0, "F1/ORPB"=0.0, "F2/ORPK"=0.0, "F3"=0.0, "F4"=0.0, "F5"=0.0, "F6"=0.0, "F7"=0.0, "X0/滴定数"=0.0, "量程"=0.0}, "关键参数改变"=FALSE, "校准信息"={"低标液1浓度"=0.0, "低标液1信号值"=0.0, "低标液1启用"=0, "低标液2浓度"=0.0, "低标液2信号值"=0.0, "低标液2启用"=0, "低标液3浓度"=0.0, "低标液3信号值"=0.0, "低标液3启用"=0, "低标液4浓度"=0.0, "低标液4信号值"=0.0, "低标液4启用"=0, "低标液5浓度"=0.0, "低标液5信号值"=0.0, "低标液5启用"=0, "高标液1浓度"=0.0, "高标液1信号值"=0.0, "高标液1启用"=0, "高标液2浓度"=0.0, "高标液2信号值"=0.0, "高标液2启用"=0, "高标液3浓度"=0.0, "高标液3信号值"=0.0, "高标液3启用"=0, "高标液4浓度"=0.0, "高标液4信号值"=0.0, "高标液4启用"=0, "高标液5浓度"=0.0, "高标液5信号值"=0.0, "高标液5启用"=0, "低斜率"=0.0, "低截距"=0.0, "低二次多项式系数"=0.0, "低线性相关系数"=0.0, "高斜率"=0.0, "高截距"=0.0, "高二次多项式系数"=0.0, "高线性相关系数"=0.0}, "校准信息改变"=FALSE, "固件版本号"=""}  # 与CODMn交互全局
      n27 = Obtain Queue(name (unnamed)="CODMn interface Read" ("写入方名称"), element data type=w56) -> (queue out=w57:refnum<queue>)  [unwired: 3 in, 2 out]
    }
  }
  n28 = case shown="True" w2 {
    tunnel: [_ w60] -> w33
    tunnel: [_ w59] -> w32
    frame False {
    }
    frame True {
      w59 = T10 {"状态告警区"={"系统时间"=timestamp(0 s since 1904-01-01), "工作状态"=0, "测量模式"=enum."待机", "告警代码"=0, "故障代码"=0, "日志代码"=0, "软件版本"=0, "F0"=0.0, "F1"=0.0, "F2"=0.0, "F3"=0.0, "T"=0.0, "H"=0.0, "id"=0, "flowid"=0, "量程"=0, "总磷控温温度1"=0.0, "营养盐控温温度2"=0.0, "ADC"=0.0}, "平台试剂余量百分比"=0.0, "关键参数"={"测量量程"=0.0, "测量精度"=0.0, "测量间隔"=0.0, "消解温度"=0.0, "消解时长"=0.0, "空白校准时间"=timestamp(0 s since 1904-01-01), "曲线截距"=0.0, "曲线斜率"=0.0, "测量检出限"=0.0, "测量信号值"=0.0, "线性相关系数"=0.0, "二次多项式系数"=0.0, "标样校准时间"=timestamp(0 s since 1904-01-01), "稀释倍数"=0.0, "三项式系数"=0.0, "空白标定系数"=0.0, "量程系数"=0.0, "F0/ORPA"=0.0, "F1/ORPB"=0.0, "F2/ORPK"=0.0, "F3"=0.0, "F4"=0.0, "F5"=0.0, "F6"=0.0, "F7"=0.0, "X0/滴定数"=0.0, "量程"=0.0}, "关键参数改变"=FALSE, "校准信息"={"低标液1浓度"=0.0, "低标液1信号值"=0.0, "低标液1启用"=0, "低标液2浓度"=0.0, "低标液2信号值"=0.0, "低标液2启用"=0, "低标液3浓度"=0.0, "低标液3信号值"=0.0, "低标液3启用"=0, "低标液4浓度"=0.0, "低标液4信号值"=0.0, "低标液4启用"=0, "低标液5浓度"=0.0, "低标液5信号值"=0.0, "低标液5启用"=0, "高标液1浓度"=0.0, "高标液1信号值"=0.0, "高标液1启用"=0, "高标液2浓度"=0.0, "高标液2信号值"=0.0, "高标液2启用"=0, "高标液3浓度"=0.0, "高标液3信号值"=0.0, "高标液3启用"=0, "高标液4浓度"=0.0, "高标液4信号值"=0.0, "高标液4启用"=0, "高标液5浓度"=0.0, "高标液5信号值"=0.0, "高标液5启用"=0, "低斜率"=0.0, "低截距"=0.0, "低二次多项式系数"=0.0, "低线性相关系数"=0.0, "高斜率"=0.0, "高截距"=0.0, "高二次多项式系数"=0.0, "高线性相关系数"=0.0}, "校准信息改变"=FALSE, "固件版本号"=""}  # 与CODCr交互全局
      n29 = Obtain Queue(name (unnamed)="CODCr interface Read" ("写入方名称"), element data type=w59) -> (queue out=w60:refnum<queue>)  [unwired: 3 in, 2 out]
    }
  }
  n30 = Not Equal?(x=w17, y=-1) -> (x != y?=w3:bool)
  n31 = Not Equal?(x=w14, y=-1) -> (x != y?=w4:bool)
  n32 = case shown="True" w4 {
    frame False {
    }
    frame True {
      n33 = call "反控参数变更.vi"("设置参数"=T9."总氮") -> ()  [unwired: 11 in]
    }
  }
  n34 = case shown="True" w3 {
    frame False {
    }
    frame True {
      n35 = call "反控参数变更.vi"("设置参数"=T9."总磷") -> ()  [unwired: 11 in]
    }
  }
  n36 = case shown="True" w5 {
    frame False {
    }
    frame True {
      n37 = call "反控参数变更.vi"("设置参数"=T9."氨氮") -> ()  [unwired: 11 in]
    }
  }
  n38 = case shown="True" w3 {
    tunnel: [_ w66] -> w31
    tunnel: [_ w65] -> w30
    frame False {
    }
    frame True {
      w65 = T11 {"状态告警区"={"系统时间"=timestamp(0 s since 1904-01-01), "工作状态"=0, "测量模式"=enum."待机", "告警代码"=0, "故障代码"=0, "日志代码"=0, "软件版本"=0, "F0"=0.0, "F1"=0.0, "F2"=0.0, "F3"=0.0, "T"=0.0, "H"=0.0, "id"=0, "flowid"=0, "量程"=0, "总磷控温温度1"=0.0, "营养盐控温温度2"=0.0, "ADC"=0.0}, "平台试剂余量百分比"=0.0, "关键参数"={"测量量程"=0.0, "测量精度"=0.0, "测量间隔"=0.0, "消解温度"=0.0, "消解时长"=0.0, "空白校准时间"=timestamp(0 s since 1904-01-01), "曲线截距"=0.0, "曲线斜率"=0.0, "测量检出限"=0.0, "测量信号值"=0.0, "线性相关系数"=0.0, "二次多项式系数"=0.0, "标样校准时间"=timestamp(0 s since 1904-01-01), "稀释倍数"=0.0, "三项式系数"=0.0, "空白标定系数"=0.0, "量程系数"=0.0, "F0/ORPA"=0.0, "F1/ORPB"=0.0, "F2/ORPK"=0.0, "F3"=0.0, "F4"=0.0, "F5"=0.0, "F6"=0.0, "F7"=0.0, "X0/滴定数"=0.0, "量程"=0.0}, "关键参数改变"=FALSE, "校准信息"={"低标液1浓度"=0.0, "低标液1信号值"=0.0, "低标液1启用"=0, "低标液2浓度"=0.0, "低标液2信号值"=0.0, "低标液2启用"=0, "低标液3浓度"=0.0, "低标液3信号值"=0.0, "低标液3启用"=0, "低标液4浓度"=0.0, "低标液4信号值"=0.0, "低标液4启用"=0, "低标液5浓度"=0.0, "低标液5信号值"=0.0, "低标液5启用"=0, "高标液1浓度"=0.0, "高标液1信号值"=0.0, "高标液1启用"=0, "高标液2浓度"=0.0, "高标液2信号值"=0.0, "高标液2启用"=0, "高标液3浓度"=0.0, "高标液3信号值"=0.0, "高标液3启用"=0, "高标液4浓度"=0.0, "高标液4信号值"=0.0, "高标液4启用"=0, "高标液5浓度"=0.0, "高标液5信号值"=0.0, "高标液5启用"=0, "低斜率"=0.0, "低截距"=0.0, "低二次多项式系数"=0.0, "低线性相关系数"=0.0, "高斜率"=0.0, "高截距"=0.0, "高二次多项式系数"=0.0, "高线性相关系数"=0.0}, "校准信息改变"=FALSE, "固件版本号"=""}  # 与总磷交互全局
      n39 = Obtain Queue(name (unnamed)="总磷 interface Read" ("写入方名称"), element data type=w65) -> (queue out=w66:refnum<queue>)  [unwired: 3 in, 2 out]
    }
  }
  n40 = case shown="True" w4 {
    tunnel: [_ w69] -> w29
    tunnel: [_ w68] -> w28
    frame False {
    }
    frame True {
      w68 = T12 {"状态告警区"={"系统时间"=timestamp(0 s since 1904-01-01), "工作状态"=0, "测量模式"=enum."待机", "告警代码"=0, "故障代码"=0, "日志代码"=0, "软件版本"=0, "F0"=0.0, "F1"=0.0, "F2"=0.0, "F3"=0.0, "T"=0.0, "H"=0.0, "id"=0, "flowid"=0, "量程"=0, "总磷控温温度1"=0.0, "营养盐控温温度2"=0.0, "ADC"=0.0}, "平台试剂余量百分比"=0.0, "关键参数"={"测量量程"=0.0, "测量精度"=0.0, "测量间隔"=0.0, "消解温度"=0.0, "消解时长"=0.0, "空白校准时间"=timestamp(0 s since 1904-01-01), "曲线截距"=0.0, "曲线斜率"=0.0, "测量检出限"=0.0, "测量信号值"=0.0, "线性相关系数"=0.0, "二次多项式系数"=0.0, "标样校准时间"=timestamp(0 s since 1904-01-01), "稀释倍数"=0.0, "三项式系数"=0.0, "空白标定系数"=0.0, "量程系数"=0.0, "F0/ORPA"=0.0, "F1/ORPB"=0.0, "F2/ORPK"=0.0, "F3"=0.0, "F4"=0.0, "F5"=0.0, "F6"=0.0, "F7"=0.0, "X0/滴定数"=0.0, "量程"=0.0}, "关键参数改变"=FALSE, "校准信息"={"低标液1浓度"=0.0, "低标液1信号值"=0.0, "低标液1启用"=0, "低标液2浓度"=0.0, "低标液2信号值"=0.0, "低标液2启用"=0, "低标液3浓度"=0.0, "低标液3信号值"=0.0, "低标液3启用"=0, "低标液4浓度"=0.0, "低标液4信号值"=0.0, "低标液4启用"=0, "低标液5浓度"=0.0, "低标液5信号值"=0.0, "低标液5启用"=0, "高标液1浓度"=0.0, "高标液1信号值"=0.0, "高标液1启用"=0, "高标液2浓度"=0.0, "高标液2信号值"=0.0, "高标液2启用"=0, "高标液3浓度"=0.0, "高标液3信号值"=0.0, "高标液3启用"=0, "高标液4浓度"=0.0, "高标液4信号值"=0.0, "高标液4启用"=0, "高标液5浓度"=0.0, "高标液5信号值"=0.0, "高标液5启用"=0, "低斜率"=0.0, "低截距"=0.0, "低二次多项式系数"=0.0, "低线性相关系数"=0.0, "高斜率"=0.0, "高截距"=0.0, "高二次多项式系数"=0.0, "高线性相关系数"=0.0}, "校准信息改变"=FALSE, "固件版本号"=""}  # 与总氮交互全局
      n41 = Obtain Queue(name (unnamed)="总氮 interface Read" ("写入方名称"), element data type=w68) -> (queue out=w69:refnum<queue>)  [unwired: 3 in, 2 out]
    }
  }
  n42 = case shown="True" w5 {
    tunnel: [_ w72] -> w27
    tunnel: [_ w71] -> w26
    frame False {
    }
    frame True {
      w71 = T13 {"状态告警区"={"系统时间"=timestamp(0 s since 1904-01-01), "工作状态"=0, "测量模式"=enum."待机", "告警代码"=0, "故障代码"=0, "日志代码"=0, "软件版本"=0, "F0"=0.0, "F1"=0.0, "F2"=0.0, "F3"=0.0, "T"=0.0, "H"=0.0, "id"=0, "flowid"=0, "量程"=0, "总磷控温温度1"=0.0, "营养盐控温温度2"=0.0, "ADC"=0.0}, "平台试剂余量百分比"=0.0, "关键参数"={"测量量程"=0.0, "测量精度"=0.0, "测量间隔"=0.0, "消解温度"=0.0, "消解时长"=0.0, "空白校准时间"=timestamp(0 s since 1904-01-01), "曲线截距"=0.0, "曲线斜率"=0.0, "测量检出限"=0.0, "测量信号值"=0.0, "线性相关系数"=0.0, "二次多项式系数"=0.0, "标样校准时间"=timestamp(0 s since 1904-01-01), "稀释倍数"=0.0, "三项式系数"=0.0, "空白标定系数"=0.0, "量程系数"=0.0, "F0/ORPA"=0.0, "F1/ORPB"=0.0, "F2/ORPK"=0.0, "F3"=0.0, "F4"=0.0, "F5"=0.0, "F6"=0.0, "F7"=0.0, "X0/滴定数"=0.0, "量程"=0.0}, "关键参数改变"=FALSE, "校准信息"={"低标液1浓度"=0.0, "低标液1信号值"=0.0, "低标液1启用"=0, "低标液2浓度"=0.0, "低标液2信号值"=0.0, "低标液2启用"=0, "低标液3浓度"=0.0, "低标液3信号值"=0.0, "低标液3启用"=0, "低标液4浓度"=0.0, "低标液4信号值"=0.0, "低标液4启用"=0, "低标液5浓度"=0.0, "低标液5信号值"=0.0, "低标液5启用"=0, "高标液1浓度"=0.0, "高标液1信号值"=0.0, "高标液1启用"=0, "高标液2浓度"=0.0, "高标液2信号值"=0.0, "高标液2启用"=0, "高标液3浓度"=0.0, "高标液3信号值"=0.0, "高标液3启用"=0, "高标液4浓度"=0.0, "高标液4信号值"=0.0, "高标液4启用"=0, "高标液5浓度"=0.0, "高标液5信号值"=0.0, "高标液5启用"=0, "低斜率"=0.0, "低截距"=0.0, "低二次多项式系数"=0.0, "低线性相关系数"=0.0, "高斜率"=0.0, "高截距"=0.0, "高二次多项式系数"=0.0, "高线性相关系数"=0.0}, "校准信息改变"=FALSE, "固件版本号"=""}  # 与氨氮交互全局
      n43 = Obtain Queue(name (unnamed)="氨氮 interface Read" ("写入方名称"), element data type=w71) -> (queue out=w72:refnum<queue>)  [unwired: 3 in, 2 out]
    }
  }
  n44 = Obtain Queue(name (unnamed)=w36, element data type=w41) -> (queue out=w37:refnum<queue>, error out=w40:errorcluster)  [unwired: 3 in, 1 out]
  n45 = Generate Occurrence() -> (w38:refnum<k4>)
  n46 = while {
    tunnel: w37 -> [w76]
    tunnel: w38 -> [w74]
    stop <- w75 stop-if-true
    n47 = event shown="[5] \"读测量数据区\": Value Change" {
      selector: _ -> [_ _ _ _ _ _ _ _]
      dyn-events: _ -> [_ _ _ _ _ _ _ _]
      timeout: _ -> [_ _ _ _ _ _ _ _]
      tunnel: w76 -> [_ _ _ w108 w118 w124 w129 w134]
      tunnel: [_ _ _ _ "停止" _ _ _] -> w75
      tunnel: w74 -> [_ _ _ _ w115 _ _ _]
      event Timeout {
        n48 = event-data() -> ()  [unwired: 1 in, 3 out]
      }
      event "启用模块": Value Change {
        n49 = event-data() -> ("NewVal"=w77:bool)  [unwired: 1 in, 5 out]
        n50 = call <vilib>:"Application Directory.vi"() -> ("Application Directory"=w79:path)
        n51 = Build Path(base path=w79, name or relative path="data\\set.ini" ("名称或相对路径")) -> (appended path=w80:path)
        n52 = call <vilib>:"Open Config Data.vi"("configuration file path"=w80) -> ("error out"=w86:errorcluster, "refnum"=w85:T14)  [unwired: 8 in, 1 out]
        n53 = call-poly <vilib>:"Write Key.vi"("section"="总磷总氮", "error in (no error)"=w86, "value"=w77, "key"="模块启用", "refnum"=w85) -> ("error out"=w82:errorcluster, "refnum out"=w78:T14)  [unwired: 4 in, 1 out]
        n54 = call <vilib>:"Close Config Data.vi"("error in (no error)"=w82, "refnum"=w78) -> ()  [unwired: 8 in, 2 out]
      }
      event "VISA Resource": Value Change {
        n55 = event-data() -> ()  [unwired: 1 in, 6 out]
        n56 = call <vilib>:"Application Directory.vi"() -> ("Application Directory"=w89:path)
        n57 = Build Path(base path=w89, name or relative path="data\\set.ini" ("名称或相对路径")) -> (appended path=w90:path)
        n58 = call <vilib>:"Open Config Data.vi"("configuration file path"=w90) -> ("error out"=w96:errorcluster, "refnum"=w95:T14)  [unwired: 8 in, 1 out]
        n59 = call-poly <vilib>:"Write Key.vi"("section"="总磷总氮", "error in (no error)"=w96, "value"="VISA Resource", "key"="串口", "refnum"=w95) -> ("error out"=w92:errorcluster, "refnum out"=w88:T14)  [unwired: 4 in, 1 out]
        n60 = call <vilib>:"Close Config Data.vi"("error in (no error)"=w92, "refnum"=w88) -> ()  [unwired: 8 in, 2 out]
      }
      event "启动": Value Change {
        n61 = event-data() -> ()  [unwired: 1 in, 6 out]
        n62 = global read "总磷总氮断电保存全局变量.vi" "协议"() -> (w99:u16)
        n63 = case shown="1" w99 {
          tunnel: "控制命令" -> [w109 w111]
          tunnel: [w109 w110] -> w97
          frame 0, Default {
          }
          frame 1 {
            n64 = Swap Bytes(anything=w111) -> (byte swapped=w110:u16)
          }
        }
        n65 = case shown="Default" "控制命令" {
          tunnel: "控制命令参数" -> [w113 w114]
          tunnel: [w112 w114] -> w100
          frame Default {
            n66 = call "HexToWord.vi"("数组"=w113) -> ("WORD"=w112:u16[])  [unwired: 10 in]
          }
          frame 13 {
          }
        }
        n67 = call "控制命令区.vi"("控制命令参数"=w100, "控制命令"=w97) -> ("控制命令"=w104:u16[])  [unwired: 9 in]
        n68 = local read "站号"() -> (w103:u16)
        n69 = Bundle("站号"=w103, "控制命令"=w104) -> (w102:cluster{"站号":u16, "控制命令":u16[]})  [unwired: 1 in]
        n70 = Bundle By Name(cluster=cluster{"命令":string, "data":variant} {"命令"="", "data"=variant} ("元素"), "命令"="启动", "data"=w102) -> (w106:cluster{"命令":string, "data":variant})
        n71 = Enqueue Element(queue=w108, element=w106) -> ()  [unwired: 2 in, 3 out]
      }
      event "停止": Value Change {
        n72 = event-data() -> ()  [unwired: 1 in, 6 out]
        n73 = Set Occurrence(w115) -> ()
        n74 = Flush Queue(queue=w118) -> (queue out=w117:refnum<queue>)  [unwired: 1 in, 2 out]
        n75 = Enqueue Element(queue=w117, element=cluster{"命令":string, "data":variant} {"命令"="shutdown", "data"=variant} ("元素")) -> ()  [unwired: 2 in, 3 out]
      }
      event "读测量数据区": Value Change {
        n76 = event-data() -> ()  [unwired: 1 in, 6 out]
        n77 = Bundle By Name(cluster=cluster{"命令":string, "data":variant} {"命令"="", "data"=variant} ("元素"), "命令"="读测量数据区", "data"="站号") -> (w122:cluster{"命令":string, "data":variant})
        n78 = Enqueue Element(queue=w124, element=w122) -> ()  [unwired: 2 in, 3 out]
      }
      event "读状态告警区": Value Change {
        n79 = event-data() -> ()  [unwired: 1 in, 6 out]
        n80 = local read "站号"() -> (w125:u16)
        n81 = Bundle By Name(cluster=cluster{"命令":string, "data":variant} {"命令"="", "data"=variant} ("元素"), "命令"="读状态告警区", "data"=w125) -> (w127:cluster{"命令":string, "data":variant})
        n82 = Enqueue Element(queue=w129, element=w127) -> ()  [unwired: 2 in, 3 out]
      }
      event "读关键参数区": Value Change {
        n83 = event-data() -> ()  [unwired: 1 in, 6 out]
        n84 = local read "站号"() -> (w130:u16)
        n85 = Bundle By Name(cluster=cluster{"命令":string, "data":variant} {"命令"="", "data"=variant} ("元素"), "命令"="读关键参数区", "data"=w130) -> (w132:cluster{"命令":string, "data":variant})
        n86 = Enqueue Element(queue=w134, element=w132) -> ()  [unwired: 2 in, 3 out]
      }
    }
  }
  n87 = while {
    tunnel: w38 -> [w145]
    tunnel: w37 -> [w141]
    stop <- w142 stop-if-true
    n88 = global read "总磷总氮断电保存全局变量.vi" "MB通信方式选择"() -> (w140:enum16{"串口", "TCP"})
    n89 = Wait on Occurrence(2:w145, 3:10000 ("毫秒超时(-1)")) -> (0:w143:bool)  [unwired: 1 in]
    n90 = Not(x=w143) -> (.not. x?=w142:bool)
    n91 = case shown="\"TCP\"" w140 {
      tunnel: [_ w146] -> w137
      frame "串口", Default {
      }
      frame "TCP" {
        n92 = global read "VAR总磷总氮全局变量.vi" "MB session in"() -> (w148:refnum<class "MB_Master.lvclass">)
        n93 = property class="MB_Master"(reference=w148) -> ("Properties:Session Valid"=w147:bool)  [unwired: 1 in, 2 out]
        n94 = Not(x=w147) -> (.not. x?=w146:bool)
      }
    }
    n95 = First Call?() -> (First Call?: T/F=w139:bool)
    n96 = Or(x=w137, y=w139) -> (x .or. y?=w138:bool)
    n97 = local read "启用"() -> (w135:bool)
    n98 = And(x=w135, y=w138) -> (x .and. y?=w136:bool)
    n99 = case shown="True" w136 {
      tunnel: w141 -> [_ w151]
      frame False {
      }
      frame True {
        n100 = Flush Queue(queue=w151) -> (queue out=w149:refnum<queue>)  [unwired: 1 in, 2 out]
        n101 = Enqueue Element(queue=w149, element=cluster{"命令":string, "data":variant} {"命令"="启用模块", "data"=variant} ("元素")) -> ()  [unwired: 2 in, 3 out]
        n102 = property on="VISA Resource" class="VISAName"("DisabledEnum"=T15."Disabled and Grayed Out" ("禁用")) -> ()  [unwired: 2 in, 2 out]
      }
    }
  }
  n103 = while {
    tunnel: w37 -> [w169]
    tunnel: w40 -> [w168]
    shift-right: [w157] -> _
    shift-left: _ -> [w166]
    tunnel: errorcluster {"status"=FALSE, "code"=0, "source"=""} ("error out") -> [w165]
    tunnel: [w154] -> _
    stop <- w167 stop-if-true
    n104 = Dequeue Element(queue=w169, error in (no error)=w168) -> (queue out=w163:refnum<queue>, element=w164:cluster{"命令":string, "data":variant})  [unwired: 1 in, 2 out]
    n105 = Unbundle By Name(w164) -> ("命令"=w153:string, "data"=w161:variant)
    n106 = case shown="\"读测量数据区\"" w153 {
      tunnel: w161 -> [_ _ _ w214 w225 w242 w245 w359 w419 _]
      tunnel: w163 -> [_ _ _ _ _ _ w248 _ _ w432]
      tunnel: [_ _ _ _ _ _ _ _ _ TRUE] -> w167
      tunnel: [w178 w181 w201 w217 w228 w244 w272 w367 w426 w428] -> w157
      tunnel: [w179 w180 w202 w216 w227 w243 w273 w358 w427 w429] -> w154
      tunnel: w166 -> [w178 _ w201 w213 w224 w241 w269 w362 w422 w428]
      tunnel: w165 -> [w179 _ w203 w210 w221 w238 w267 w363 w423 w430]
      tunnel: [_ _ _ w205 w218 w232 w250 w340 w413 _] -> w155
      frame Default {
      }
      frame "启用模块" {
        n107 = global read "总磷总氮断电保存全局变量.vi" "MB通信方式选择"() -> (w182:enum16{"串口", "TCP"})
        n108 = case shown="\"串口\", Default" w182 {
          tunnel: [w192 w197] -> w180
          tunnel: [w190 w196] -> w181
          frame "串口", Default {
            n109 = global read "总磷总氮断电保存全局变量.vi" "VISA Resource"() -> (w185:refnum<visa-resource-name>)
            n110 = global read "总磷总氮断电保存全局变量.vi" "波特率"() -> (w188:u32)
            n111 = VISA Close(VISA resource name=w185) -> (error out=w186:errorcluster)  [unwired: 1 in]
            n112 = Bundle By Name(cluster=T16 {"baud rate (bps)"=115200, "stop bits"=10, "parity"=0, "flow control"=0, "timeout"=1000, "retries"=1} ("Serial Config"), "baud rate (bps)"=w188) -> (w187:T16)
            n113 = call <vilib>:"Clear Errors.vi"("error in (no error)"=w186) -> ("error out"=w184:errorcluster)  [unwired: 5 in, 1 out]
            n114 = call <vilib>:"Open Serial Session.vi"("Mode (RTU)"=enum16{"RTU", "ASCII"}."RTU", "Error in"=w184, "Slave ID"=u8 1, "Serial Config"=w187, "VISA Resource"=w185) -> ("Error out"=w192:errorcluster, "MB_Serial session"=w190:refnum<class "MB_Master_Serial.lvclass">)  [unwired: 5 in]
          }
          frame "TCP" {
            n115 = global read "总磷总氮断电保存全局变量.vi" "PORT"() -> (w195:string)
            n116 = Decimal String To Number(string=w195) -> (number=w198:i32)  [unwired: 2 in, 1 out]
            n117 = global read "总磷总氮断电保存全局变量.vi" "IP"() -> (w194:string)
            n118 = call <vilib>:"Open TCP Session.vi"("Port (502)"=w198, "IP Address"=w194) -> ("error out"=w197:errorcluster, "MB_TCP session"=w196:refnum<class "MB_Master_TCP.lvclass">)  [unwired: 8 in]
          }
        }
        "启用" <- TRUE
      }
      frame "停用模块" {
        n119 = call-dynamic "Close Session.vi"("error in (no error)"=w203, "MB session in"=w201) -> ("error out"=w199:errorcluster)  [unwired: 9 in]
        n120 = local write "启用"(FALSE ("启用")) -> ()
        n121 = call <vilib>:"Clear Errors.vi"("error in (no error)"=w199) -> ("error out"=w202:errorcluster)  [unwired: 5 in, 1 out]
      }
      frame "启动" {
        n122 = Variant To Data(type=cluster{"站号":u16, "控制命令":u16[]} {"站号"=0, "控制命令"=[]} ("输出簇"), Variant=w214) -> (data=w208:cluster{"站号":u16, "控制命令":u16[]})  [unwired: 1 in, 1 out]
        n123 = Unbundle By Name(w208) -> ("站号"=w205:u16, "控制命令"=w206:u16[])
        n124 = property class="MB_Master"(reference=w213, error in=w210, "Properties:Slave ID"=w205) -> (reference out=w212:refnum<class "MB_Master.lvclass">, error out=w211:errorcluster)
        n125 = Index Array(array=w206) -> (element=w207:u16)  [unwired: 1 in]
        n126 = Swap Bytes(anything=w207) -> (byte swapped=w204:u16)
        n127 = global write "VAR总磷总氮全局变量.vi" "控制命令"(w204) -> ()
        n128 = call <vilib>:"Write Multiple Registers.vi"("error in (no error)"=w211, "values"=w206, "starting address"=u16 4608, "MB session in"=w212) -> ("error out"=w216:errorcluster, "MB session out"=w217:refnum<class "MB_Master.lvclass">)  [unwired: 6 in]
      }
      frame "盲样测试" {
        n129 = Variant To Data(type=u8 0, Variant=w225) -> (data=w218:u8)  [unwired: 1 in, 1 out]
        n130 = property class="MB_Master"(reference=w224, error in=w221, "Properties:Slave ID"=w218) -> (reference out=w223:refnum<class "MB_Master.lvclass">, error out=w222:errorcluster)
        n131 = case shown="3" w218 {
          tunnel: [u16[] [] ("values") u16[] [33539, 0] ("values") u16[] [23555, 0] ("values")] -> w220
          frame Default {
          }
          frame 1 {
            # "总磷盲样测试命令"
          }
          frame 3 {
            # "氨氮盲样测试"
          }
        }
        n132 = call <vilib>:"Write Multiple Registers.vi"("error in (no error)"=w222, "values"=w220, "starting address"=u16 24592, "MB session in"=w223) -> ("error out"=w227:errorcluster, "MB session out"=w228:refnum<class "MB_Master.lvclass">)  [unwired: 6 in]
      }
      frame "debug" {
        n133 = Variant To Data(type=cluster{"站号":u16, "控制命令":u16[]} {"站号"=0, "控制命令"=[]} ("输出簇"), Variant=w242) -> (data=w236:cluster{"站号":u16, "控制命令":u16[]})  [unwired: 1 in, 1 out]
        n134 = Unbundle By Name(w236) -> ("站号"=w232:u16, "控制命令"=w234:u16[])
        n135 = property class="MB_Master"(reference=w241, error in=w238, "Properties:Slave ID"=w232) -> (reference out=w240:refnum<class "MB_Master.lvclass">, error out=w239:errorcluster)
        n136 = Index Array(array=w234) -> (element=w235:u16)  [unwired: 1 in]
        n137 = global write "VAR总磷总氮全局变量.vi" "控制命令"(w235) -> ()
        n138 = call <vilib>:"Write Multiple Registers.vi"("error in (no error)"=w239, "values"=w234, "starting address"=u16 24594, "MB session in"=w240) -> ("error out"=w243:errorcluster, "MB session out"=w244:refnum<class "MB_Master.lvclass">)  [unwired: 6 in]
      }
      frame "读测量数据区" {
        n139 = Variant To Data(type=u8 1 ("Slave ID"), Variant=w245) -> (data=w250:u8)  [unwired: 1 in, 1 out]
        n140 = property class="MB_Master"(reference=w269, error in=w267, "Properties:Slave ID"=w250) -> (reference out=w268:refnum<class "MB_Master.lvclass">, error out=w266:errorcluster)
        n141 = Bundle("命令"="读关键参数区", "data"=w245) -> (w246:cluster{"命令":string, "data":variant})  [unwired: 1 in]
        n142 = global read "VAR总磷总氮全局变量.vi" "测量数据区数组"() -> (w263:T8)
        n143 = call "id参数转换.vi"("id"=w250) -> ("数组资源索引"=w259:i32)  [unwired: 9 in, 1 out]
        n144 = Enqueue Element(queue=w248, element=w246) -> ()  [unwired: 2 in, 3 out]
        n145 = call <vilib>:"Read Holding Registers.vi"("error in (no error)"=w266, "quantity"=u16 107, "starting address"=u16 4096, "MB session in"=w268) -> ("error out"=w273:errorcluster, "Registers"=w265:u16[], "MB session out"=w272:refnum<class "MB_Master.lvclass">)  [unwired: 5 in]
        n146 = call "id参数转换.vi"("id"=u16 2) -> ("数组资源索引"=w256:i32)  [unwired: 9 in, 1 out]
        n147 = call "id参数转换.vi"("id"=u16 3) -> ("数组资源索引"=w254:i32)  [unwired: 9 in, 1 out]
        n148 = Index Array(array=w263, index #1=w259, index #2=w256, index #3=w254) -> (element #1=w264:T5, element #2=w260:T5, element #3=w258:T5)
        n149 = call "测量数据区_选择.vi"("Slave ID"=w250, "data"=w265) -> ("测量数据区"=w251:T5)  [unwired: 9 in]
        "测量数据区" <- w251
        n150 = global write "VAR总磷总氮全局变量.vi" "测量数据区"(w251) -> ()
        n151 = global read "工况数据接口全局.vi" "data"() -> (w253:T17)
        n152 = case shown="2" w250 {
          tunnel: w251 -> [w275 w282 w323 w331 w338]
          tunnel: w265 -> [_ w295 w324 w332 w339]
          tunnel: w264 -> [_ w288 _ _ _]
          tunnel: [w275 w290 w323 w331 w338] -> w262
          tunnel: w260 -> [_ w286 _ _ _]
          tunnel: w258 -> [_ w285 _ _ _]
          tunnel: w253 -> [w274 w283 w322 w330 w337]
          tunnel: [w274 w276 w311 w325 w336] -> w252
          tunnel: w251 -> [_ _ w321 w329 w335]
          frame 0, Default {
          }
          frame 1 {
            n153 = Unbundle By Name(w282) -> ("F0"=w281:sgl, "F1"=w280:sgl, "F2"=w279:sgl, "F3"=w278:sgl, "X值"=w277:sgl)
            n154 = Bundle By Name(cluster=w283, "data.TP.TP.F0"=w281, "data.TP.TP.F1"=w280, "data.TP.TP.F2"=w279, "data.TP.TP.F3"=w278, "data.TP.TP.X0"=w277) -> (w276:T17)
            n155 = global read "VAR总磷总氮全局变量.vi" "模块名称"() -> (w294:string)
            n156 = Search and Replace String(input string=w294, search string="总磷" ("搜索字符串")) -> (result string=w291:string, offset past replacement=w292:i32)  [unwired: 6 in, 2 out]
            n157 = case shown="Default" w292 {
              tunnel: w291 -> [_ w301]
              tunnel: [_ w298] -> w289
              tunnel: [_ w296] -> w287
              frame -1 {
              }
              frame Default {
                n158 = Search and Replace String(input string=w301, search string="总氮" ("搜索字符串")) -> (offset past replacement=w304:i32)  [unwired: 6 in, 3 out]
                n159 = Search and Replace String(input string=w301, search string="氨氮" ("搜索字符串")) -> (offset past replacement=w299:i32)  [unwired: 6 in, 3 out]
                n160 = Not Equal?(x=w304, y=-1) -> (x != y?=w296:bool)
                n161 = Not Equal?(x=w299, y=-1) -> (x != y?=w297:bool)
                n162 = Or(x=w297, y=w296) -> (x .or. y?=w298:bool)
              }
            }
            n163 = Select(t=w286, s=w287, f=w285) -> (s? t:f=w284:T5)
            n164 = case shown="True" w289 {
              tunnel: [w306 w310] -> w290
              tunnel: w288 -> [_ w309]
              tunnel: w284 -> [_ w308]
              tunnel: w282 -> [w306 w307]
              frame False {
              }
              frame True {
                # "启动总磷总氮时间自动对齐"
                n165 = call "数据时间对齐.vi"("待对齐时间"=w307, "对齐参考时间"=w308, "已对齐时间输入"=w309) -> ("已对齐时间输出"=w310:T5)  [unwired: 8 in]
              }
            }
            "总磷测量数据区" <- w295
          }
          frame 2 {
            n166 = Unbundle By Name(w321) -> ("F0"=w320:sgl, "F1"=w319:sgl, "F2"=w318:sgl, "F3"=w317:sgl, "F4"=w316:sgl, "F5"=w315:sgl, "F6"=w314:sgl, "F7"=w313:sgl, "X值"=w312:sgl)
            n167 = Bundle By Name(cluster=w322, "data.TN.TN.F0"=w320, "data.TN.TN.F1"=w319, "data.TN.TN.F2"=w318, "data.TN.TN.F3"=w317, "data.TN.TN.F4"=w316, "data.TN.TN.F5"=w315, "data.TN.TN.F6"=w314, "data.TN.TN.F7"=w313, "data.TN.TN.X0"=w312) -> (w311:T17)
            "总氮测量数据区" <- w324
          }
          frame 3 {
            n168 = Unbundle By Name(w329) -> ("F0"=w328:sgl, "F1"=w327:sgl, "X值"=w326:sgl)
            n169 = Bundle By Name(cluster=w330, "data.NH3.NH3.F0"=w328, "data.NH3.NH3.F1"=w327, "data.NH3.NH3.X0"=w326) -> (w325:T17)
            "氨氮测量数据区" <- w332
          }
          frame 22 {
            n170 = Unbundle By Name(w335) -> ("F0"=w334:sgl, "F1"=w333:sgl)
            n171 = Bundle By Name(cluster=w337, "data.CODCr.CODCr.F0"=w334, "data.CODCr.CODCr.F1"=w333) -> (w336:T17)
            "COD测量数据区" <- w339
          }
        }
        n172 = global write "工况数据接口全局.vi" "data"(w252) -> ()
        n173 = Replace Array Subset(array=w263, new element=w262, index=w259) -> (w261:T8)
        n174 = global write "VAR总磷总氮全局变量.vi" "测量数据区数组"(w261) -> ()
      }
      frame "读状态告警区" {
        n175 = Variant To Data(type=u8 1 ("Slave ID"), Variant=w359) -> (data=w340:u8)  [unwired: 1 in, 1 out]
        n176 = property class="MB_Master"(reference=w362, error in=w363, "Properties:Slave ID"=w340) -> (reference out=w361:refnum<class "MB_Master.lvclass">, error out=w360:errorcluster)
        n177 = call "id参数转换.vi"("id"=w340) -> ("数组资源索引"=w353:i32)  [unwired: 9 in, 1 out]
        n178 = call <vilib>:"Read Holding Registers.vi"("error in (no error)"=w360, "quantity"=u16 44, "starting address"=u16 4224, "MB session in"=w361) -> ("error out"=w358:errorcluster, "Registers"=w356:u16[], "MB session out"=w367:refnum<class "MB_Master.lvclass">)  [unwired: 5 in]
        n179 = global read "VAR总磷总氮全局变量.vi" "状态告警区数组"() -> (w355:T7)
        n180 = call "状态告警区_选择.vi"("data"=w356) -> ("状态告警区 2"=w341:T18, "状态告警区"=w342:T4)  [unwired: 9 in]
        "状态告警区" <- w341
        n181 = Unbundle By Name(w342) -> ("日志代码"=w343:u16, "告警代码"=w349:u16, "故障代码"=w347:u16)
        n182 = global write "VAR总磷总氮全局变量.vi" "状态告警区"(w341) -> ()
        n183 = Unbundle By Name(w342) -> ("id"=w357:u16)
        n184 = Replace Array Subset(array=w355, new element=w342, index=w353) -> (w354:T7)
        n185 = global write "VAR总磷总氮全局变量.vi" "状态告警区数组"(w354) -> ()
        n186 = feedback-in #1(w349) -> ()
        n187 = feedback #1() -> (w350:u16)  [unwired: 1 in]
        n188 = feedback #2() -> (w348:u16)  [unwired: 1 in]
        n189 = feedback-in #2(w347) -> ()
        n190 = Not Equal?(x=w350, y=w349) -> (x != y?=w346:bool)
        n191 = Not Equal?(x=w348, y=w347) -> (x != y?=w345:bool)
        n192 = Or(x=w346, y=w345) -> (x .or. y?=w344:bool)
        n193 = global read "工况数据接口全局.vi" "data"() -> (w352:T17)
        n194 = case shown="1, 131" w357 {
          tunnel: w342 -> [_ w380 w393 w403 w409]
          tunnel: w356 -> [_ w381 w394 w404 w411]
          tunnel: w352 -> [w368 w371 w386 w399 w410]
          tunnel: [w368 w378 w388 w402 w407] -> w351
          tunnel: w344 -> [_ w373 w384 w398 _]
          tunnel: w343 -> [_ w372 w383 w397 _]
          frame 0, Default {
          }
          frame 1, 131 {
            n195 = Unbundle By Name(w371) -> ("data.TP.TP.alarm_step"=w370:dbl)
            n196 = Unbundle By Name(w380) -> ("总磷控温温度1"=w379:sgl, "营养盐控温温度2"=w375:sgl)
            n197 = Select(t=w372, s=w373, f=w370) -> (s? t:f=w369:dbl)
            n198 = global read "VAR总磷总氮全局变量.vi" "总磷关键参数"() -> (w377:T19)
            n199 = Unbundle By Name(w377) -> ("消解温度"=w376:sgl)
            n200 = Bundle By Name(cluster=w371, "data.TP.TP.alarm_step"=w369, "data.TP.TP.digestion_temperature"=w379, "data.TP.TP.constant_temperature"=w376, "data.TP.TP.syringe_temperature"=w375, "data.TP.启用"=TRUE) -> (w378:T17)
            "总磷状态告警区" <- w381
          }
          frame 2, 76 {
            n201 = Unbundle By Name(w386) -> ("data.TN.TN.alarm_step"=w385:dbl)
            n202 = Unbundle By Name(w393) -> ("总磷控温温度1"=w389:sgl, "营养盐控温温度2"=w391:sgl)
            n203 = Select(t=w383, s=w384, f=w385) -> (s? t:f=w382:dbl)
            n204 = global read "VAR总磷总氮全局变量.vi" "总氮关键参数"() -> (w392:T19)
            n205 = Unbundle By Name(w392) -> ("消解温度"=w390:sgl)
            n206 = Bundle By Name(cluster=w386, "data.TN.TN.alarm_step"=w382, "data.TN.TN.digestion_temperature"=w389, "data.TN.TN.constant_temperature"=w390, "data.TN.TN.syringe_temperature"=w391, "data.TN.启用"=TRUE) -> (w388:T17)
            "总氮状态告警区" <- w394
          }
          frame 3 {
            n207 = Unbundle By Name(w399) -> ("data.NH3.NH3.alarm_step"=w396:dbl)
            n208 = Unbundle By Name(w403) -> ("营养盐控温温度2"=w401:sgl)
            n209 = Select(t=w397, s=w398, f=w396) -> (s? t:f=w395:dbl)
            n210 = Bundle By Name(cluster=w399, "data.NH3.NH3.alarm_step"=w395, "data.NH3.NH3.syringe_temperature"=w401, "data.NH3.启用"=TRUE) -> (w402:T17)
            "氨氮状态告警区" <- w404
          }
          frame 22 {
            n211 = Unbundle By Name(w409) -> ("营养盐控温温度2"=w408:sgl)
            n212 = global read "VAR总磷总氮全局变量.vi" "波形图-消解温度"() -> (w405:sgl[])
            n213 = Bundle By Name(cluster=w410, "data.CODCr.CODCr.temperature_curve"=w405, "data.CODCr.CODCr.reagent_sensor"=w408, "data.CODCr.启用"=TRUE) -> (w407:T17)
            "COD状态告警区" <- w411
          }
        }
        n214 = global write "工况数据接口全局.vi" "data"(w351) -> ()
      }
      frame "读关键参数区" {
        n215 = Variant To Data(type=u8 1 ("Slave ID"), Variant=w419) -> (data=w413:u8)  [unwired: 1 in, 1 out]
        n216 = property class="MB_Master"(reference=w422, error in=w423, "Properties:Slave ID"=w413) -> (reference out=w421:refnum<class "MB_Master.lvclass">, error out=w420:errorcluster)
        n217 = call "id参数转换.vi"("id"=w413) -> ("数组资源索引"=w412:i32)  [unwired: 9 in, 1 out]
        n218 = call <vilib>:"Read Holding Registers.vi"("error in (no error)"=w420, "quantity"=u16 56, "starting address"=u16 4256, "MB session in"=w421) -> ("error out"=w427:errorcluster, "Registers"=w417:u16[], "MB session out"=w426:refnum<class "MB_Master.lvclass">)  [unwired: 5 in]
        n219 = global read "VAR总磷总氮全局变量.vi" "关键参数区数组"() -> (w416:T6)
        n220 = call "关键参数区.vi"("数组"=w417) -> ("关键参数区"=w415:T20)  [unwired: 10 in]
        "关键参数区" <- w415
        n221 = global write "VAR总磷总氮全局变量.vi" "关键参数区"(w415) -> ()
        n222 = Replace Array Subset(array=w416, new element=w415, index=w412) -> (w414:T6)
        n223 = global write "VAR总磷总氮全局变量.vi" "关键参数区数组"(w414) -> ()
      }
      frame "shutdown" {
        n224 = call-dynamic "Close Session.vi"("error in (no error)"=w430, "MB session in"=w428) -> ("error out"=w429:errorcluster)  [unwired: 9 in]
        n225 = Flush Queue(queue=w432) -> (queue out=w431:refnum<queue>)  [unwired: 1 in, 2 out]
        n226 = Release Queue(queue=w431) -> ()  [unwired: 2 in, 3 out]
      }
    }
    n227 = disable-structure shown="禁用" {
      disable-tunnel: w154 -> [w171 _]
      disable-tunnel: w153 -> [w170 _]
      frame Disabled {
        n228 = case shown="Error" w171 {
          selector: w171 -> [_ w175]
          tunnel: w170 -> [_ w174]
          frame No Error {
          }
          frame Error {
            n229 = Unbundle By Name(w175) -> ("source"=w173:string)
            n230 = Concatenate Strings(w174, w173) -> (w172:string)
            n231 = One Button Dialog(message=w172) -> ()  [unwired: 1 in, 1 out]
          }
        }
      }
      frame Enabled {
      }
    }
    n232 = global write "VAR总磷总氮全局变量.vi" "MB session in"(w157) -> ()
    n233 = Unbundle By Name(w154) -> ("status"=w160:bool)
    n234 = Not(x=w160) -> (.not. x?=w162:bool)
    "status" <- w162
    n235 = call <vilib>:"Boolean Crossing PtByPt.vi"("direction"=enum16{"either", "false-true", "true-false"}."false-true", "input"=w160) -> ("crossing"=w159:bool)  [unwired: 1 in]
    n236 = case shown="True" w159 {
      tunnel: [u16 0 ("告警代码") u16 999 ("告警代码")] -> w156
      frame False {
      }
      frame True {
      }
    }
    n237 = global write "VAR总磷总氮全局变量.vi" "通讯状态"(w162) -> ()
    n238 = call "告警码字段定义.vi"("id"=w155, "告警代码"=w156) -> ()  [unwired: 9 in, 1 out]
  }
  n239 = while {
    tunnel: w35 -> [w444]
    tunnel: w34 -> [w443]
    tunnel: w33 -> [w442]
    tunnel: w32 -> [w441]
    tunnel: w31 -> [w440]
    tunnel: w30 -> [w439]
    tunnel: w29 -> [w438]
    tunnel: w28 -> [w437]
    tunnel: w27 -> [w436]
    tunnel: w26 -> [w435]
    stop <- FALSE stop-if-true
    n240 = global read "model config var.vi" "启动队列名称"() -> (w447:cluster{"String":string, "Value":u16}[])
    n241 = Wait (ms)(milliseconds to wait=u32 1000 ("等待时间（毫秒）")) -> ()  [unwired: 1 out]
    n242 = global read "VAR总磷总氮全局变量.vi" "固件版本号"() -> (w434:string)
    n243 = for {
      tunnel: w447 -> [w460] mode=indexing
      tunnel: w444 -> [w458]
      tunnel: w443 -> [w457]
      tunnel: w442 -> [w456]
      tunnel: w441 -> [w455]
      tunnel: w440 -> [w454]
      tunnel: w439 -> [w453]
      tunnel: w438 -> [w452]
      tunnel: w437 -> [w451]
      tunnel: w436 -> [w450]
      tunnel: w435 -> [w449]
      tunnel: w434 -> [w448]
      n244 = Unbundle By Name(w460) -> ("Value"=w459:u16)
      n245 = case shown="22" w459 {
        tunnel: w458 -> [_ _ _ _ w547 _]
        tunnel: w457 -> [_ _ _ _ w546 _]
        tunnel: w456 -> [_ _ _ w526 _ _]
        tunnel: w455 -> [_ _ _ w525 _ _]
        tunnel: w454 -> [w463 _ _ _ _ _]
        tunnel: w453 -> [w462 _ _ _ _ _]
        tunnel: w452 -> [_ w484 _ _ _ _]
        tunnel: w451 -> [_ w483 _ _ _ _]
        tunnel: w450 -> [_ _ w505 _ _ _]
        tunnel: w449 -> [_ _ w504 _ _ _]
        tunnel: w448 -> [w461 w482 w503 w524 w545 _]
        frame 1 {
          n246 = Get Queue Status(queue=w463) -> (queue out=w466:refnum<queue>, # elements in queue=w465:i32)  [unwired: 2 in, 6 out]
          n247 = Equal To 0?(x=w465) -> (x = 0?=w464:bool)
          n248 = case shown="True" w464 {
            tunnel: w462 -> [_ w478]
            tunnel: w466 -> [_ w479]
            tunnel: w461 -> [_ w467]
            frame False {
            }
            frame True {
              w469 = u16 1 items=["总磷"=1, "总氮"=2, "氨氮"=3, "磷酸盐"=4, "硝氮"=5, "亚硝氮"=6, "硅酸盐"=7, "硫化物"=8, "CODCr"=22]
              n249 = Unbundle By Name(w478) -> ("关键参数"=w476:T21)
              n250 = global read "VAR总磷总氮全局变量.vi" "总磷关键参数"() -> (w477:T19)
              n251 = global read "VAR总磷总氮全局变量.vi" "状态告警区数组"() -> (w471:T7)
              n252 = global read "VAR总磷总氮全局变量.vi" "平台试剂余量百分比"() -> (w481:sgl)
              n253 = call "id参数转换.vi"("id"=w469) -> ("数组资源索引"=w470:i32)  [unwired: 9 in, 1 out]
              n254 = call "转换关键参数(子VI).vi"("参数"=w469, "总磷关键参数"=w477, "关键参数输入"=w476) -> ("关键参数输出"=w475:T21)  [unwired: 8 in]
              n255 = global read "VAR总磷总氮全局变量.vi" "总磷关键参数改变"() -> (w474:bool)
              n256 = global read "VAR总磷总氮全局变量.vi" "总磷校准信息改变"() -> (w472:bool)
              n257 = global read "VAR总磷总氮全局变量.vi" "总磷校准信息"() -> (w473:T22)
              n258 = Index Array(array=w471, index=w470) -> (element=w468:T4)
              n259 = Bundle By Name(cluster=w478, "状态告警区"=w468, "平台试剂余量百分比"=w481, "关键参数"=w475, "关键参数改变"=w474, "校准信息"=w473, "校准信息改变"=w472, "固件版本号"=w467) -> (w480:T11)
              n260 = Enqueue Element(queue=w479, element=w480) -> ()  [unwired: 2 in, 3 out]
            }
          }
        }
        frame 2 {
          n261 = Get Queue Status(queue=w484) -> (queue out=w487:refnum<queue>, # elements in queue=w486:i32)  [unwired: 2 in, 6 out]
          n262 = Equal To 0?(x=w486) -> (x = 0?=w485:bool)
          n263 = case shown="True" w485 {
            tunnel: w487 -> [_ w500]
            tunnel: w483 -> [_ w498]
            tunnel: w482 -> [_ w488]
            frame False {
            }
            frame True {
              w490 = u16 2 items=["总磷"=1, "总氮"=2, "氨氮"=3, "磷酸盐"=4, "硝氮"=5, "亚硝氮"=6, "硅酸盐"=7, "硫化物"=8, "CODCr"=22]
              n264 = Unbundle By Name(w498) -> ("关键参数"=w497:T21)
              n265 = global read "VAR总磷总氮全局变量.vi" "总氮关键参数"() -> (w499:T19)
              n266 = global read "VAR总磷总氮全局变量.vi" "状态告警区数组"() -> (w491:T7)
              n267 = global read "VAR总磷总氮全局变量.vi" "平台试剂余量百分比"() -> (w502:sgl)
              n268 = call "id参数转换.vi"("id"=w490) -> ("数组资源索引"=w492:i32)  [unwired: 9 in, 1 out]
              n269 = call "转换关键参数(子VI).vi"("参数"=w490, "总磷关键参数"=w499, "关键参数输入"=w497) -> ("关键参数输出"=w496:T21)  [unwired: 8 in]
              n270 = global read "VAR总磷总氮全局变量.vi" "总氮关键参数改变"() -> (w495:bool)
              n271 = global read "VAR总磷总氮全局变量.vi" "总氮校准信息改变"() -> (w493:bool)
              n272 = global read "VAR总磷总氮全局变量.vi" "总氮校准信息"() -> (w494:T22)
              n273 = Index Array(array=w491, index=w492) -> (element=w489:T4)
              n274 = Bundle By Name(cluster=w498, "状态告警区"=w489, "平台试剂余量百分比"=w502, "关键参数"=w496, "关键参数改变"=w495, "校准信息"=w494, "校准信息改变"=w493, "固件版本号"=w488) -> (w501:T12)
              n275 = Enqueue Element(queue=w500, element=w501) -> ()  [unwired: 2 in, 3 out]
            }
          }
        }
        frame 3 {
          (unwired) FALSE
          n276 = Get Queue Status(queue=w505) -> (queue out=w507:refnum<queue>, # elements in queue=w508:i32)  [unwired: 2 in, 6 out]
          n277 = Equal To 0?(x=w508) -> (x = 0?=w506:bool)
          n278 = case shown="True" w506 {
            tunnel: w507 -> [_ w521]
            tunnel: w504 -> [_ w520]
            tunnel: w503 -> [_ w509]
            frame False {
            }
            frame True {
              w511 = u16 3 items=["总磷"=1, "总氮"=2, "氨氮"=3, "磷酸盐"=4, "硝氮"=5, "亚硝氮"=6, "硅酸盐"=7, "硫化物"=8, "CODCr"=22]
              n279 = Unbundle By Name(w520) -> ("关键参数"=w519:T21)
              n280 = global read "VAR总磷总氮全局变量.vi" "氨氮关键参数"() -> (w517:T19)
              n281 = global read "VAR总磷总氮全局变量.vi" "状态告警区数组"() -> (w512:T7)
              n282 = global read "VAR总磷总氮全局变量.vi" "平台试剂余量百分比"() -> (w523:sgl)
              n283 = call "id参数转换.vi"("id"=w511) -> ("数组资源索引"=w513:i32)  [unwired: 9 in, 1 out]
              n284 = call "转换关键参数(子VI).vi"("参数"=w511, "总磷关键参数"=w517, "关键参数输入"=w519) -> ("关键参数输出"=w518:T21)  [unwired: 8 in]
              n285 = global read "VAR总磷总氮全局变量.vi" "氨氮关键参数改变"() -> (w516:bool)
              n286 = global read "VAR总磷总氮全局变量.vi" "氨氮校准信息改变"() -> (w514:bool)
              n287 = global read "VAR总磷总氮全局变量.vi" "氨氮校准信息"() -> (w515:T22)
              n288 = Index Array(array=w512, index=w513) -> (element=w510:T4)
              n289 = Bundle By Name(cluster=w520, "状态告警区"=w510, "平台试剂余量百分比"=w523, "关键参数"=w518, "关键参数改变"=w516, "校准信息"=w515, "校准信息改变"=w514, "固件版本号"=w509) -> (w522:T13)
              n290 = Enqueue Element(queue=w521, element=w522) -> ()  [unwired: 2 in, 3 out]
            }
          }
        }
        frame 22 {
          n291 = Get Queue Status(queue=w526) -> (queue out=w528:refnum<queue>, # elements in queue=w529:i32)  [unwired: 2 in, 6 out]
          n292 = Equal To 0?(x=w529) -> (x = 0?=w527:bool)
          n293 = case shown="True" w527 {
            tunnel: w528 -> [_ w542]
            tunnel: w525 -> [_ w541]
            tunnel: w524 -> [_ w530]
            frame False {
            }
            frame True {
              w532 = u16 22 items=["总磷"=1, "总氮"=2, "氨氮"=3, "磷酸盐"=4, "硝氮"=5, "亚硝氮"=6, "硅酸盐"=7, "硫化物"=8, "CODCr"=22]
              n294 = Unbundle By Name(w541) -> ("关键参数"=w540:T21)
              n295 = global read "VAR总磷总氮全局变量.vi" "CODcr关键参数"() -> (w539:T19)
              n296 = global read "VAR总磷总氮全局变量.vi" "状态告警区数组"() -> (w533:T7)
              n297 = global read "VAR总磷总氮全局变量.vi" "CODCr关键参数改变"() -> (w537:bool)
              n298 = global read "VAR总磷总氮全局变量.vi" "CODCr校准信息改变"() -> (w535:bool)
              n299 = global read "VAR总磷总氮全局变量.vi" "平台试剂余量百分比"() -> (w544:sgl)
              n300 = call "id参数转换.vi"("id"=w532) -> ("数组资源索引"=w534:i32)  [unwired: 9 in, 1 out]
              n301 = call "转换关键参数(子VI).vi"("参数"=w532, "总磷关键参数"=w539, "关键参数输入"=w540) -> ("关键参数输出"=w538:T21)  [unwired: 8 in]
              n302 = global read "VAR总磷总氮全局变量.vi" "CODCr校准信息"() -> (w536:T22)
              n303 = Index Array(array=w533, index=w534) -> (element=w531:T4)
              n304 = Bundle By Name(cluster=w541, "状态告警区"=w531, "平台试剂余量百分比"=w544, "关键参数"=w538, "关键参数改变"=w537, "校准信息"=w536, "校准信息改变"=w535, "固件版本号"=w530) -> (w543:T10)
              n305 = Enqueue Element(queue=w542, element=w543) -> ()  [unwired: 2 in, 3 out]
            }
          }
        }
        frame 21 {
          (unwired) FALSE
          n306 = Get Queue Status(queue=w547) -> (queue out=w549:refnum<queue>, # elements in queue=w550:i32)  [unwired: 2 in, 6 out]
          n307 = Equal To 0?(x=w550) -> (x = 0?=w548:bool)
          n308 = case shown="True" w548 {
            tunnel: w549 -> [_ w563]
            tunnel: w546 -> [_ w562]
            tunnel: w545 -> [_ w551]
            frame False {
            }
            frame True {
              w553 = u16 21 items=["总磷"=1, "总氮"=2, "氨氮"=3, "磷酸盐"=4, "硝氮"=5, "亚硝氮"=6, "硅酸盐"=7, "硫化物"=8, "CODMn"=21, "CODCr"=22, "氟化物"=50]
              n309 = Unbundle By Name(w562) -> ("关键参数"=w561:T21)
              n310 = global read "VAR总磷总氮全局变量.vi" "CODMn关键参数"() -> (w560:T19)
              n311 = global read "VAR总磷总氮全局变量.vi" "状态告警区数组"() -> (w554:T7)
              n312 = global read "VAR总磷总氮全局变量.vi" "CODmn关键参数改变"() -> (w558:bool)
              n313 = global read "VAR总磷总氮全局变量.vi" "CODMn校准信息改变"() -> (w556:bool)
              n314 = global read "VAR总磷总氮全局变量.vi" "平台试剂余量百分比"() -> (w565:sgl)
              n315 = call "id参数转换.vi"("id"=w553) -> ("数组资源索引"=w555:i32)  [unwired: 9 in, 1 out]
              n316 = call "转换关键参数(子VI).vi"("参数"=w553, "总磷关键参数"=w560, "关键参数输入"=w561) -> ("关键参数输出"=w559:T21)  [unwired: 8 in]
              n317 = global read "VAR总磷总氮全局变量.vi" "CODMn校准信息"() -> (w557:T22)
              n318 = Index Array(array=w554, index=w555) -> (element=w552:T4)
              n319 = Bundle By Name(cluster=w562, "状态告警区"=w552, "平台试剂余量百分比"=w565, "关键参数"=w559, "关键参数改变"=w558, "校准信息"=w557, "校准信息改变"=w556, "固件版本号"=w551) -> (w564:T10)
              n320 = Enqueue Element(queue=w563, element=w564) -> ()  [unwired: 2 in, 3 out]
            }
          }
        }
        frame Default {
        }
      }
    }
  }
  n321 = flat-sequence {
    tunnel: [w567] -> w8
    frame #0 {
      n322 = Wait (ms)(milliseconds to wait=u32 10000 ("等待时间（毫秒）")) -> ()  [unwired: 1 out]
    }
    frame #1 {
      n323 = global read "model config var.vi" "启动队列名称"() -> (w567:cluster{"String":string, "Value":u16}[])
    }
  }
  n324 = for {
    tunnel: w8 -> [w574] mode=indexing
    tunnel: [w569] -> w7 mode=indexing
    tunnel: [w568] -> w6 mode=indexing
    n325 = Unbundle By Name(w574) -> ("String"=w570:string)
    n326 = Concatenate Strings(w570, "固件升级" ("字符串")) -> (w572:string)
    n327 = Obtain Queue(name (unnamed)=w572, element data type=cluster{"selected path":path} {"selected path"=path ""}) -> (queue out=w569:refnum<queue>, error out=w568:errorcluster)  [unwired: 3 in, 1 out]
  }
  n328 = while {
    tunnel: w7 -> [w579]
    tunnel: w6 -> [w578]
    tunnel: [w577] -> _
    tunnel: [w576] -> _
    stop <- FALSE stop-if-true
    n329 = for {
      tunnel: w579 -> [w586] mode=indexing
      tunnel: w578 -> [w585] mode=indexing
      tunnel: [w584] -> w577
      tunnel: [w583] -> w576
      n330 = Dequeue Element(queue=w586, timeout in ms (-1)=1000 ("超时毫秒(-1)"), error in (no error)=w585) -> (queue out=w584:refnum<queue>, element=w582:cluster{"selected path":path}, timed out?=w580:bool, error out=w583:errorcluster)
      n331 = case shown="False" w580 {
        tunnel: w582 -> [w595 _]
        frame False {
          n332 = Unbundle By Name(w595) -> ("selected path"=w594:path)
          n333 = call "固件升级（包含参数恢复）.vi"("路径对话框"=FALSE, "selected path"=w594) -> ("结果字符串"=w588:string)  [unwired: 9 in]
          n334 = global read "VAR总磷总氮全局变量.vi" "模块名称"() -> (w590:string)
          n335 = Concatenate Strings("平台反控固件升级" ("日志信息"), w588) -> (w587:string)
          n336 = Get Date/Time In Seconds() -> (seconds since 1Jan1904=w591:timestamp)
          n337 = Bundle By Name(cluster=T23 {"时间"=timestamp(0 s since 1904-01-01), "参数"="", "日志信息"="", "流程参数"=""} ("data in"), "时间"=w591, "参数"=w590, "日志信息"=w587) -> (w592:T23)
          n338 = call "总磷总氮操作日志.vi"("data in"=w592) -> ()  [unwired: 10 in, 1 out]
        }
        frame True {
        }
      }
    }
  }
